vi "Saccade.vi"() -> ()   [LabVIEW 2012]
uses:
  <vilib>/Platform/TimedLoop/XDataNode/timing_clust.ctl
  <vilib>/Platform/TimedLoop/XDataNode/nitl_modes.ctl
  <vilib>/Platform/TimedLoop/XDataNode/wakeup.ctl
  <vilib>/DAQmx/write.llb/DAQmx Write (Analog DBL 1Chan 1Samp).vi
  <vilib>/DAQmx/miscellaneous.llb/DAQmx Fill In Error Info.vi
  SubVIs/VariablesToString_String.vi
  SubVIs/VariablesToString_Scalar.vi
  <vilib>/Platform/TimedLoop/XDataNode/XDataNode.xnode
  <vilib>/Platform/TimedLoop/XDataNode/XDNodeRunTimeDep.lvlib
  <vilib>/nisyscfg/nisyscfg.lvlib
  <vilib>/DAQmx/write.llb/DAQmx Write (Digital 1D Bool NChan 1Samp 1Line).vi
panel:
  in  "WfFlag":bool=TRUE
  out "WfGraph":cluster{dbl, dbl, dbl[][]}(graph)={-0.35, 0.04, array2x7714[15428 elements]}
  in  "SAFlag":bool
  in  "ElecStimSettings":T1={"TL"=200.0, "Freq"=200.0, "Dur"=0.2, "Amp"=10.0, "TD"=0.0, "DState"=enum."Ground", "TL2"=200.0, "Freq2"=200.0, "Dur2"=0.2, "Amp2"=10.0, "TD2"=0.0} {"Amp2" min=0.0 max=100.0 step=5.0; "Freq2" min=25.0 max=500.0 step=25.0; "Amp" min=0.0 max=100.0 step=5.0; "Freq" min=25.0 max=500.0 step=25.0}
  out "TrialStatus":T2={"TrialState"=enum."Initialize", "InitializeState"=enum."0", "FinalizeState"=enum."0", "HandsStatus"=enum."Both Hands On", "StimType"=enum."Photic", "Outcome"=enum."Abort", "AbortReason"=enum."Timed Out", "AbortLocation"=enum."Acq Stimulus"}
  out "GetHostTimeVI":path=path "E:/Code/Tasks/SubVIs/GetHostTime.vi"
  out "RunProgramVI":path=path "E:/Code/Tasks/SubVIs/RunProgram.vi"
  out "StopRecording":bool
  out "SaccadeFolder":path=path "E:/Code/Tasks/Saccade/Saccade_v2.0"
  out "CerebusFolder":string
  out "Recording?":bool
  out "AutoCentraVI":path=path "E:/Code/Tasks/SubVIs/AutoCentral.vi"
  out "TaskType":string="Saccade.vi"
  out "DatabaseUDL":path=path "E:/Data/Setup1_Database.udl"
  in  "Database":T3={"ExperimentDate"=timestamp(-9593222400 s since 1904-01-01), "ImplantDate"=timestamp(-9593222400 s since 1904-01-01), "CerebusFolder"="", "Experimenter"="", "PatientNumber"="", "DominantHand"="", "DeviceType"="", "DeviceSerial"="", "DeviceHemisphere"="", "DeviceRegion"="", "TaskType"="", "TaskComments"="", "RecordingComments"="", "GeneralObservations"=""}
  out "RemotePort":u16=9500
  out "RemoteIP":u32=2607134730
  out "UDPRef":refnum<k16>
  in  "RandFlag":bool
  in  "PhoticBnds":enum16{"Full Field", "LR Quadrant"}(ring)=enum."LR Quadrant" caption="Photic Bounds"
  out "AbortCount":u64
  in  "PlotSaccades":bool=TRUE
  out "LastPhoticStimPresets":T4(radio)=enum."Selection 1" caption="Stimulus Position"
  out "EyeXY":dbl[](array[numeric])=[0.6988403336972048, 0.026813536037091617] caption="Eye Position (X/Y)" format="%#.1g"
  out "EyeStatus":T5={"Fixation"=enum."In", "Photic"=enum."Out", "Electric"=enum."Out"}
  in  "SetElec":bool
  in  "ElectrodeStr":string="16;17;18;19,20,26;27;28;29,30,36;37;38;39;40;46;47;48;49;50;56;57;58;59;60;\r16;17;18;19;20;26;27;28;29;30;36;37;38;39;40;46;47;48;49,50,56;57;58;59,60,\r"
  out "ElectricArray":dbl[][](array[numeric])
  out "PhoticArray":dbl[][](array[numeric])
  in  "RandPhotic":bool
  out "Finished Late? [i-1]":bool
  out "ExpTime":u32 caption="Timer (min)" max=48 step=1
  out "Time/Date":timestamp=timestamp(3443552991.074658 s since 1904-01-01) format="%<%X\n%m/%d/%Y>T"
  out "LoopPeriod":u64=2
  out "LoopCount":u64=29507
  in  "StimSwitchSettings":T6={"ElecStimMode"=enum."Manual", "ElecPerc"=0.1}
  out "Damage Plot":cluster{"Y":dbl[], "Y":dbl[]}[](graph)=[{"Y"=[50.0], "Y"=[2.4999999999999996]}, {"Y"=[100.0, 0.0], "Y"=[0.0, 5.0]}] caption="Elec Curve"
  out "Current Electrode":i32=19 caption="Electrode"
  in  "RecordsSelection":string(combo)
  out "ExperimentDate":timestamp
  out "StimTypeBigIndicator":enum32{"---", "Photic", "Electric"}(ring)=enum."Photic" caption="Stimulation Type"
  out "MATLABCom":string="LV.ID='DrawPStim';LV.StimX=4.00;LV.StimY=0.00;LV.Radius=0.15;LV.Intensity=0.10;"
  out "LEDs":T7
  in  "ArrayReset":bool
  in  "Elec Indicators":T8={"Pulse Current"=250.0, "Pulse Charge"=50.0, "Pulse Charge Density"=2.4999999999999996, "SurfaceArea"=2000.0, "PhaseDuration"=0.2} {"PhaseDuration" format="%.4g"; "SurfaceArea" format="%.4g"; "Pulse Charge Density" format="%.4g"; "Pulse Charge" format="%.4g"; "Pulse Current" format="%.4g"}
  in  "Electrodes":T9={"Mixed Checkbox"=enum."False", "Mixed Checkbox 2"=enum."False", "Mixed Checkbox 3"=enum."False", "Mixed Checkbox 4"=enum."False", "Mixed Checkbox 5"=enum."False", "Mixed Checkbox 6"=enum."False", "Mixed Checkbox 7"=enum."False", "Mixed Checkbox 8"=enum."False", "Mixed Checkbox 9"=enum."False", "Mixed Checkbox 10"=enum."False", "Mixed Checkbox 11"=enum."False", "Mixed Checkbox 12"=enum."False", "Mixed Checkbox 13"=enum."False", "Mixed Checkbox 14"=enum."False", "Mixed Checkbox 15"=enum."False", "Mixed Checkbox 16"=enum."Mixed", "Mixed Checkbox 17"=enum."Mixed", "Mixed Checkbox 18"=enum."Mixed", "Mixed Checkbox 19"=enum."True", "Mixed Checkbox 20"=enum."True", "Mixed Checkbox 21"=enum."False", "Mixed Checkbox 22"=enum."False", "Mixed Checkbox 23"=enum."False", "Mixed Checkbox 24"=enum."False", "Mixed Checkbox 25"=enum."False", "Mixed Checkbox 26"=enum."Mixed", "Mixed Checkbox 27"=enum."Mixed", "Mixed Checkbox 28"=enum."Mixed", "Mixed Checkbox 29"=enum."True", "Mixed Checkbox 30"=enum."True", "Mixed Checkbox 31"=enum."False", "Mixed Checkbox 32"=enum."False", "Mixed Checkbox 33"=enum."False", "Mixed Checkbox 34"=enum."False", "Mixed Checkbox 35"=enum."False", "Mixed Checkbox 36"=enum."Mixed", "Mixed Checkbox 37"=enum."Mixed", "Mixed Checkbox 38"=enum."Mixed", "Mixed Checkbox 39"=enum."Mixed", "Mixed Checkbox 40"=enum."Mixed", "Mixed Checkbox 41"=enum."False", "Mixed Checkbox 42"=enum."False", "Mixed Checkbox 43"=enum."False", "Mixed Checkbox 44"=enum."False", "Mixed Checkbox 45"=enum."False", "Mixed Checkbox 46"=enum."Mixed", "Mixed Checkbox 47"=enum."Mixed", "Mixed Checkbox 48"=enum."Mixed", "Mixed Checkbox 49"=enum."Mixed", "Mixed Checkbox 50"=enum."Mixed", "Mixed Checkbox 51"=enum."False", "Mixed Checkbox 52"=enum."False", "Mixed Checkbox 53"=enum."False", "Mixed Checkbox 54"=enum."False", "Mixed Checkbox 55"=enum."False", "Mixed Checkbox 56"=enum."Mixed", "Mixed Checkbox 57"=enum."Mixed", "Mixed Checkbox 58"=enum."Mixed", "Mixed Checkbox 59"=enum."Mixed", "Mixed Checkbox 60"=enum."Mixed", "Mixed Checkbox 61"=enum."False", "Mixed Checkbox 62"=enum."False", "Mixed Checkbox 63"=enum."False", "Mixed Checkbox 64"=enum."False", "Mixed Checkbox 65"=enum."False", "Mixed Checkbox 66"=enum."False", "Mixed Checkbox 67"=enum."False", "Mixed Checkbox 68"=enum."False", "Mixed Checkbox 69"=enum."False", "Mixed Checkbox 70"=enum."False", "Mixed Checkbox 71"=enum."False", "Mixed Checkbox 72"=enum."False", "Mixed Checkbox 73"=enum."False", "Mixed Checkbox 74"=enum."False", "Mixed Checkbox 75"=enum."False", "Mixed Checkbox 76"=enum."False", "Mixed Checkbox 77"=enum."False", "Mixed Checkbox 78"=enum."False", "Mixed Checkbox 79"=enum."False", "Mixed Checkbox 80"=enum."False", "Mixed Checkbox 81"=enum."False", "Mixed Checkbox 82"=enum."False", "Mixed Checkbox 83"=enum."False", "Mixed Checkbox 84"=enum."False", "Mixed Checkbox 85"=enum."False", "Mixed Checkbox 86"=enum."False", "Mixed Checkbox 87"=enum."False", "Mixed Checkbox 88"=enum."False", "Mixed Checkbox 89"=enum."False", "Mixed Checkbox 90"=enum."False", "Mixed Checkbox 91"=enum."False", "Mixed Checkbox 92"=enum."False", "Mixed Checkbox 93"=enum."False", "Mixed Checkbox 94"=enum."False", "Mixed Checkbox 95"=enum."False", "Mixed Checkbox 96"=enum."False", "Mixed Checkbox 97"=enum."False", "Mixed Checkbox 98"=enum."False", "Mixed Checkbox 99"=enum."False", "Mixed Checkbox 100"=enum."False"}
  in  "StimButton":bool
  in  "PauseControls":T10={"Stimulate"=FALSE, "StimLoad"=FALSE, "Fixate"=FALSE, "PauseType"=FALSE, "FixationTime"=500.0}
  in  "Global Controls":T11={"Stop"=FALSE, "Pause"=FALSE, "TrackEyes"=TRUE, "MonHands"=FALSE, "Comment"=FALSE, "ElecReset"=FALSE, "PhoticReset"=FALSE}
  in  "Timers":T12={"ST"={"AFD"=2000, "SD"=1000, "HF"=2000, "HS"=1000, "BRD"=350, "FPD"=1000, "AS"=1000}, "RT"={"AFD"=0, "SD"=0, "HF"=300, "HS"=0, "BRD"=100, "AS"=0, "FPD"=100}, "AT"={"AFD"=2000, "SD"=300, "HF"=2105, "HS"=1000, "BRD"=282, "AS"=1000, "FPD"=907}} {"RT"."FPD" step=1; "RT"."AS" step=1; "RT"."SD" step=1; "RT"."AFD" step=1; "RT"."HF" step=1; "RT"."HS" step=1; "RT"."BRD" step=1; "AT"."FPD" max=1000 step=50; "AT"."AS" max=10000 step=100; "AT"."SD" max=10000 step=100; "AT"."AFD" max=10000 step=100; "AT"."HF" max=10000 step=50; "AT"."HS" max=10000 step=100; "AT"."BRD" max=1000 step=50; "ST"."FPD" step=1; "ST"."SD" step=1; "ST"."AFD" step=1; "ST"."HF" step=1; "ST"."HS" step=1; "ST"."BRD" step=1; "ST"."AS" step=1}
  in  "PhoticStimSettings":T13={"StimIntensity"=0.1, "StimRadius"=0.15, "StimX"=4.0, "StimY"=0.0, "BGnd"=0.0} caption="Photic Stimulus Settings" {"BGnd" format="%.2f"; "StimIntensity" format="%.3g"; "StimRadius" min=0.1 max=1.0 format="%.2g"; "StimY" format="%.2f"; "StimX" format="%.2f"}
  out "Stats":T14={"Photic"={"AcqStimulus"=7.0, "HoldStimulus"=0.0, "HoldFixation"=0.0, "Successful"=0.0, "Total"=7.0, "RemovedHands"=0.0}, "Electric"={"AcqStimulus"=2.0, "HoldStimulus"=0.0, "HoldFixation"=0.0, "Successful"=0.0, "Total"=2.0, "RemovedHands"=0.0}} {"Electric"."RemovedHands" min=0.0 format="%#.4g"; "Electric"."Total" min=0.0 format="%#.4g"; "Electric"."Successful" min=0.0 format="%#.4g"; "Electric"."HoldFixation" min=0.0 format="%#.4g"; "Electric"."HoldStimulus" min=0.0 format="%#.4g"; "Electric"."AcqStimulus" min=0.0 format="%#.4g"; "Photic"."RemovedHands" min=0.0 format="%#.4g"; "Photic"."Total" min=0.0 format="%#.4g"; "Photic"."Successful" min=0.0 format="%#.4g"; "Photic"."HoldFixation" min=0.0 format="%#.4g"; "Photic"."HoldStimulus" min=0.0 format="%#.4g"; "Photic"."AcqStimulus" min=0.0 format="%#.4g"}
  in  "PhoticStimPresets":T4(radio)=enum."Selection 1" caption="Stimulus Position"
  in  "EyeCalibration":T15={"Eye"={"OffsetX"=-0.6000000000000002, "OffsetY"=0.9000000000000005, "GainNegX"=5.279999999999999, "GainNegY"=4.1000000000000005, "GainPosX"=6.1, "GainPosY"=3.920000000000007, "RotNegX"=0.039999999999999994, "RotNegY"=0.0, "RotPosX"=-0.039999999999999994, "RotPosY"=0.12000000000000209}, "Fix"={"X"=0.0, "Y"=0.0, "R"=1.5}, "Photic"={"X"=4.0, "Y"=0.0, "R"=1.4999999999999998}, "Elec"={"X"=5.550000000000005, "Y"=-6.000000000000007, "R"=4.000000000000011}} caption="Eye Calibration" {"Elec"."X" min=-100.0 max=100.0 step=0.05 format="%.2f"; "Elec"."Y" min=-100.0 max=100.0 step=0.05 format="%.2f"; "Elec"."R" min=-100.0 max=100.0 step=0.05 format="%.2g"; "Photic"."X" min=-100.0 max=100.0 step=0.05 format="%.2f"; "Photic"."Y" min=-100.0 max=100.0 step=0.05 format="%.2f"; "Photic"."R" min=-100.0 max=100.0 step=0.05 format="%.2g"; "Fix"."X" min=-100.0 max=100.0 step=0.05 format="%.2f"; "Fix"."Y" min=-100.0 max=100.0 step=0.05 format="%.2f"; "Fix"."R" min=-100.0 max=100.0 step=0.05 format="%.2g"; "Eye"."RotPosY" min=-100.0 max=100.0 step=0.02 format="%.2g"; "Eye"."RotPosX" min=-100.0 max=100.0 step=0.02 format="%.2f"; "Eye"."RotNegY" min=-100.0 max=100.0 step=0.02 format="%.2g"; "Eye"."RotNegX" min=-100.0 max=100.0 step=0.02 format="%.2f"; "Eye"."GainPosY" min=-100.0 max=100.0 step=0.02 format="%.2g"; "Eye"."GainPosX" min=-100.0 max=100.0 step=0.02 format="%.2f"; "Eye"."GainNegY" min=-100.0 max=100.0 step=0.02 format="%.2g"; "Eye"."GainNegX" min=-100.0 max=100.0 step=0.02 format="%.2f"; "Eye"."OffsetY" min=-100.0 max=100.0 step=0.02 format="%.2g"; "Eye"."OffsetX" min=-100.0 max=100.0 step=0.02 format="%.2g"}
  out "Eye Graph":cluster{"Y":dbl[], "Y":dbl[]}[](graph)=[{"Y"=[0.6988403336972048], "Y"=[0.026813536037091617]}, {"Y"=[], "Y"=[]}, {"Y"=[0.0, 0.1879998503464564, 0.37303483074728216, 0.5521868290270169, 0.722630511152573, 0.8816778784387097, 1.0268206588930329, 1.155769864163684, 1.2664918882530225, 1.3572405786990294, 1.4265847744427302, 1.4734308760930328, 1.4970400926424072, 1.4970400926424072, 1.473430876093033, 1.4265847744427305, 1.3572405786990291, 1.2664918882530225, 1.155769864163684, 1.0268206588930333, 0.8816778784387098, 0.7226305111525728, 0.5521868290270172, 0.37303483074728283, 0.1879998503464568, 1.836909530733566e-16, -0.18799985034645644, -0.37303483074728183, -0.5521868290270169, -0.722630511152573, -0.881677878438709, -1.0268206588930326, -1.155769864163684, -1.266491888253023, -1.3572405786990296, -1.4265847744427302, -1.473430876093033, -1.4970400926424072, -1.4970400926424072, -1.473430876093033, -1.4265847744427305, -1.3572405786990298, -1.2664918882530225, -1.1557698641636844, -1.0268206588930333, -0.88167787843871, -0.7226305111525742, -0.5521868290270168, -0.37303483074728305, -0.18799985034645697, -3.673819061467132e-16], "Y"=[1.5, 1.4881720519717168, 1.4528747416929466, 1.3946647288323772, 1.3144600200657954, 1.2135254915624212, 1.0934529411321172, 0.9561359846230346, 0.8037401924684948, 0.638668937347609, 0.4635254915624212, 0.2810719718785871, 0.09418577929397029, -0.0941857792939701, -0.2810719718785869, -0.4635254915624207, -0.6386689373476091, -0.8037401924684953, -0.9561359846230346, -1.093452941132117, -1.213525491562421, -1.3144600200657954, -1.394664728832377, -1.4528747416929464, -1.4881720519717168, -1.5, -1.4881720519717168, -1.4528747416929468, -1.3946647288323772, -1.3144600200657952, -1.2135254915624216, -1.0934529411321177, -0.9561359846230343, -0.8037401924684945, -0.6386689373476082, -0.46352549156242134, -0.28107197187858696, -0.09418577929396982, 0.09418577929396925, 0.2810719718785864, 0.46352549156242084, 0.6386689373476078, 0.8037401924684952, 0.956135984623034, 1.0934529411321168, 1.213525491562421, 1.3144600200657948, 1.3946647288323772, 1.4528747416929464, 1.4881720519717168, 1.5]}, {"Y"=[4.0, 4.187999850346456, 4.373034830747282, 4.552186829027017, 4.722630511152573, 4.88167787843871, 5.026820658893033, 5.155769864163684, 5.2664918882530225, 5.357240578699029, 5.4265847744427305, 5.473430876093033, 5.497040092642408, 5.497040092642408, 5.473430876093033, 5.4265847744427305, 5.357240578699029, 5.2664918882530225, 5.155769864163684, 5.026820658893033, 4.88167787843871, 4.722630511152572, 4.552186829027017, 4.373034830747283, 4.187999850346457, 4.0, 3.8120001496535436, 3.6269651692527183, 3.4478131709729833, 3.277369488847427, 3.118322121561291, 2.9731793411069676, 2.844230135836316, 2.7335081117469775, 2.6427594213009704, 2.57341522555727, 2.526569123906967, 2.5029599073575928, 2.5029599073575928, 2.526569123906967, 2.5734152255572695, 2.6427594213009704, 2.7335081117469775, 2.844230135836316, 2.9731793411069667, 3.11832212156129, 3.277369488847426, 3.4478131709729833, 3.626965169252717, 3.812000149653543, 3.9999999999999996], "Y"=[1.4999999999999998, 1.4881720519717165, 1.4528747416929464, 1.394664728832377, 1.3144600200657952, 1.213525491562421, 1.0934529411321172, 0.9561359846230345, 0.8037401924684947, 0.6386689373476089, 0.4635254915624211, 0.28107197187858707, 0.09418577929397028, -0.09418577929397008, -0.28107197187858685, -0.4635254915624206, -0.638668937347609, -0.8037401924684952, -0.9561359846230345, -1.0934529411321168, -1.2135254915624207, -1.3144600200657952, -1.3946647288323768, -1.4528747416929462, -1.4881720519717165, -1.4999999999999998, -1.4881720519717165, -1.4528747416929466, -1.394664728832377, -1.314460020065795, -1.2135254915624214, -1.0934529411321174, -0.9561359846230342, -0.8037401924684944, -0.6386689373476081, -0.4635254915624213, -0.2810719718785869, -0.09418577929396979, 0.09418577929396924, 0.28107197187858635, 0.4635254915624208, 0.6386689373476077, 0.803740192468495, 0.9561359846230338, 1.0934529411321168, 1.2135254915624207, 1.3144600200657945, 1.394664728832377, 1.4528747416929462, 1.4881720519717165, 1.4999999999999998]}, {"Y"=[], "Y"=[]}, {"Y"=[5.550000000000005, 6.051332934257223, 6.544759548659427, 7.022498210738721, 7.477014696406871, 7.901141009169904, 8.288188423714766, 8.632052971103171, 8.927311702008074, 9.169308209864093, 9.35422606518063, 9.47914900291477, 9.542106913713102, 9.542106913713102, 9.47914900291477, 9.35422606518063, 9.169308209864093, 8.927311702008074, 8.632052971103171, 8.288188423714768, 7.901141009169905, 7.477014696406871, 7.022498210738721, 6.544759548659429, 6.051332934257225, 5.550000000000006, 5.048667065742786, 4.555240451340584, 4.077501789261289, 3.6229853035931385, 3.198858990830108, 2.8118115762852445, 2.4679470288968397, 2.172688297991935, 1.9306917901359162, 1.7457739348193808, 1.6208509970852396, 1.5578930862869083, 1.5578930862869083, 1.6208509970852396, 1.7457739348193804, 1.9306917901359157, 2.1726882979919364, 2.467947028896839, 2.8118115762852423, 3.1988589908301055, 3.6229853035931354, 4.07750178926129, 4.555240451340581, 5.0486670657427855, 5.550000000000004], "Y"=[-1.9999999999999964, -2.031541194742085, -2.1256673554854726, -2.2808940564469915, -2.4947732798245434, -2.763932022500209, -3.0841254903143533, -3.4503040410052415, -3.856692820084015, -4.296882833739712, -4.763932022500214, -5.250474741657106, -5.748837921882752, -6.251162078117261, -6.749525258342907, -7.236067977499799, -7.703117166260302, -8.143307179916, -8.549695958994773, -8.91587450968566, -9.236067977499804, -9.505226720175472, -9.719105943553021, -9.874332644514542, -9.968458805257928, -10.000000000000018, -9.96845880525793, -9.874332644514542, -9.719105943553023, -9.50522672017547, -9.236067977499808, -8.915874509685661, -8.549695958994771, -8.143307179915999, -7.7031171662603, -7.2360679774998005, -6.749525258342907, -6.251162078117261, -5.748837921882755, -5.250474741657108, -4.763932022500215, -4.296882833739716, -3.8566928200840143, -3.4503040410052432, -3.0841254903143547, -2.7639320225002093, -2.494773279824545, -2.2808940564469915, -2.125667355485473, -2.0315411947420854, -1.9999999999999964]}, {"Y"=[], "Y"=[]}, {"Y"=[], "Y"=[]}, {"Y"=[0.0], "Y"=[0.0]}, {"Y"=[], "Y"=[]}, {"Y"=[4.0], "Y"=[0.0]}, {"Y"=[], "Y"=[]}, {"Y"=[5.550000000000005], "Y"=[-6.000000000000007]}, {"Y"=[], "Y"=[]}, {"Y"=[], "Y"=[]}, {"Y"=[3.5, 7.5, 7.5, 3.5, 3.5], "Y"=[-5.0, -5.0, -7.0, -7.0, -5.0]}, {"Y"=[6.0, -1.1021457184401395e-15, 9.0, 8.314915792601582, 3.44415089128581, -1.6532185776602093e-15, 12.0, 11.086554390135442, 8.485281374238568, 4.59220118838108, -2.204291436880279e-15], "Y"=[0.0, -6.0, 0.0, -3.444150891285806, -8.31491579260158, -9.0, 0.0, -4.5922011883810745, -8.485281374238571, -11.08655439013544, -12.0]}]
  in  "Comments":string="Stimming the six groups of 9."
  out "ExpStartTime":u32=96660144
  # "Global Controls"
  # "Eye Tracking Graph"
  # "Trial Parameters"
  # "Electric Parameters"
  # "Database"
  # "Electrodes"
  # "1  2  3  4  5  6  7  8  9 10"
  # "0  1  2  3  4  5  6  7  8  9"
  # "0  1  2  3  4  5  6  7  8  9"
  # "Wire Bundle"
  # "Photic Parameters"
  # "1  2  3  4  5  6  7  8  9 10"
  # "Eye Calibration"
  # "Pulse Parameters"
  # "Status Panel"
  # "Damage Threshold"
  # "Statistics"
  # "Do not place ';' or '=' in the comment fields"
  # "Pause Controls"
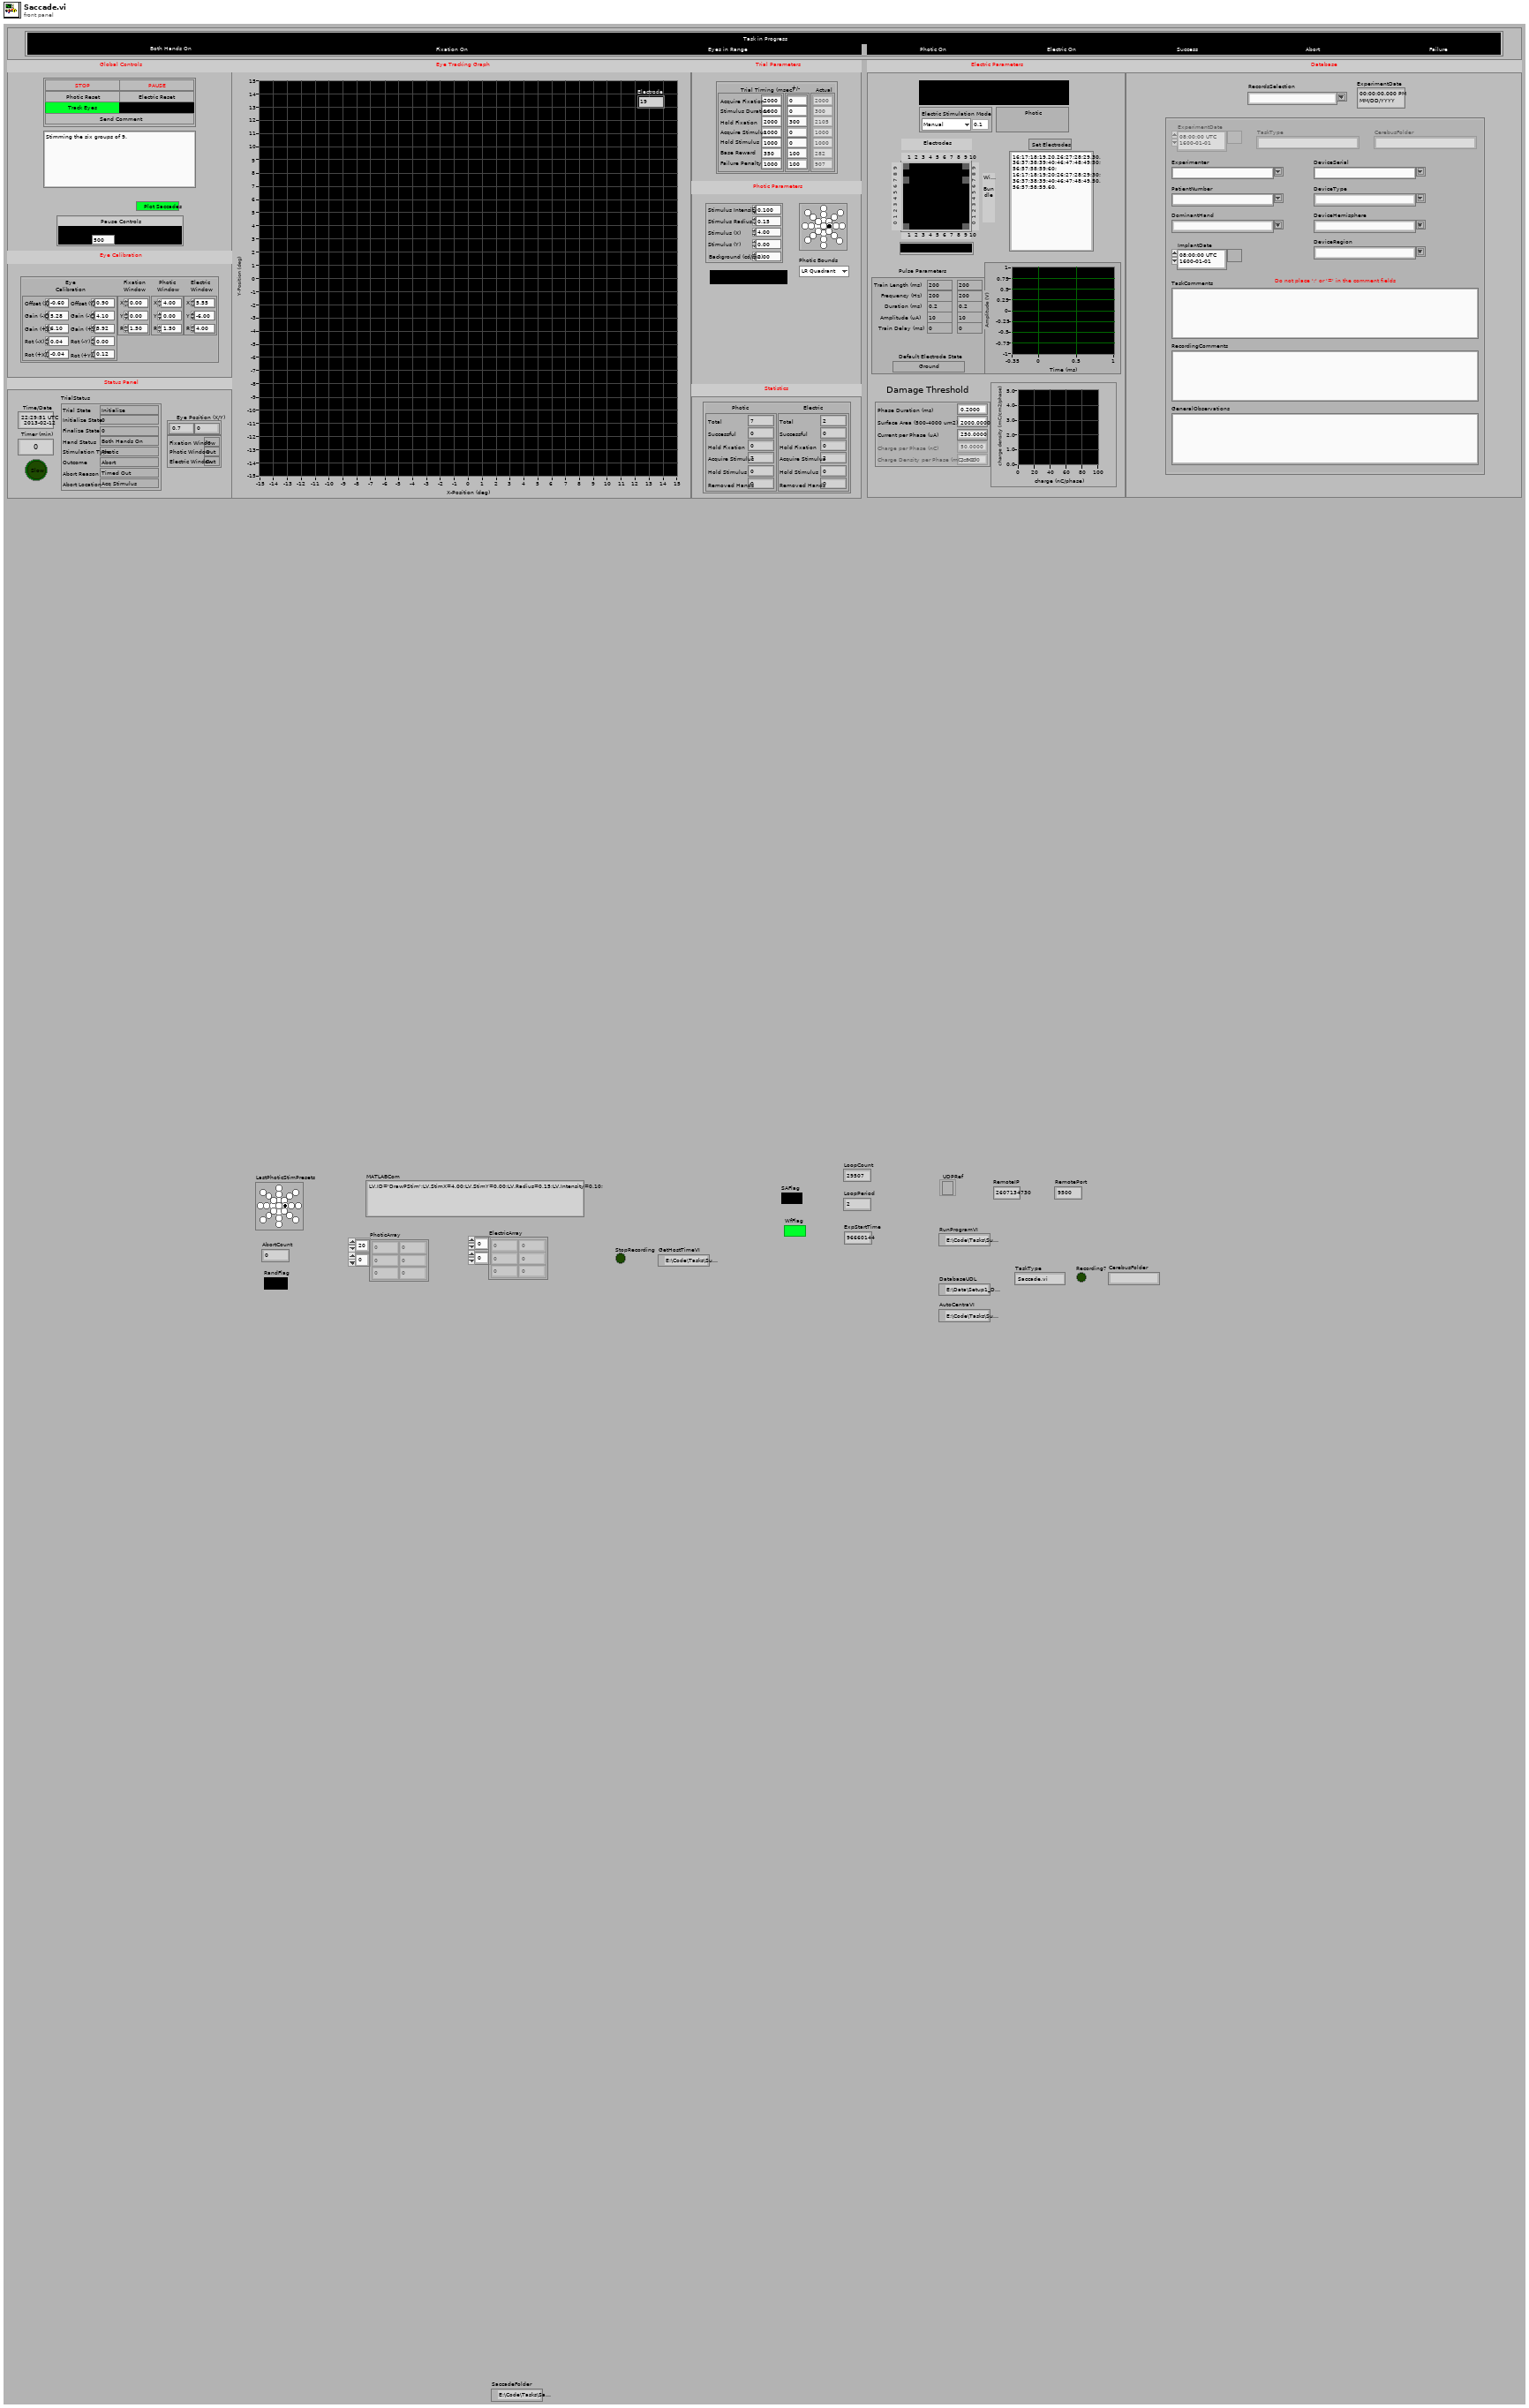
[diagram p1: front panel]
types:
  T1 = cluster{"TL":dbl, "Freq":dbl, "Dur":dbl, "Amp":dbl, "TD":dbl, "DState":enum16{"Ground", "Zero Current", "Open"}, "TL2":dbl, "Freq2":dbl, "Dur2":dbl, "Amp2":dbl, "TD2":dbl}
  T2 = cluster{"TrialState":enum32{"Initialize", "Acquire Fixation", "Visual Stimuli", "Finalize"}, "InitializeState":enum32{"0", "1", "2", "3", "4", "5", "6", "7", "8", "9", "10"}, "FinalizeState":enum32{"0", "1", "2", "3", "4", "5", "6", "7", "8", "9", "10"}, "HandsStatus":enum32{"Both Hands Off", "Left Hand Off", "Right Hand Off", "Both Hands On"}, "StimType":enum32{"---", "Photic", "Electric"}, "Outcome":enum32{"---", "Success", "Abort"}, "AbortReason":enum32{"---", "Looked Away", "Removed Hands", "Timed Out"}, "AbortLocation":enum32{"---", "Visual Stimuli", "Hold Fixation", "Acq Stimulus", "Hold Stimulus"}}
  T3 = cluster{"ExperimentDate":timestamp, "ImplantDate":timestamp, "CerebusFolder":string, "Experimenter":string, "PatientNumber":string, "DominantHand":string, "DeviceType":string, "DeviceSerial":string, "DeviceHemisphere":string, "DeviceRegion":string, "TaskType":string, "TaskComments":string, "RecordingComments":string, "GeneralObservations":string}
  T4 = enum32{"Selection 0", "Selection 1", "Selection 2", "Selection 3", "Selection 4", "Selection 5", "Selection 6", "Selection 7", "Selection 8", "Selection 9", "Selection 10", "Selection 11", "Selection 12", "Selection 13", "Selection 14", "Selection 15", "Selection 16", "Selection 17", "Selection 18", "Selection 19", "Selection 20", "Selection 21", "Selection 22", "Selection 23", "Selection 24"}
  T5 = cluster{"Fixation":enum16{"In", "Out"}, "Photic":enum16{"In", "Out"}, "Electric":enum16{"In", "Out"}}
  T6 = cluster{"ElecStimMode":enum16{"Continuous", "Manual"}, "ElecPerc":dbl}
  T7 = cluster{"InRange":bool, "TaskInProgress":bool, "Fixation":bool, "PStim":bool, "Success":bool, "Failure":bool, "Abort":bool, "HandsReady":bool, "RightHand":bool, "LeftHand":bool, "EStim":bool}
  T8 = cluster{"Pulse Current":dbl, "Pulse Charge":dbl, "Pulse Charge Density":dbl, "SurfaceArea":dbl, "PhaseDuration":dbl}
  T9 = cluster{"Mixed Checkbox":enum8{"False", "True", "Mixed"}, "Mixed Checkbox 2":enum8{"False", "True", "Mixed"}, "Mixed Checkbox 3":enum8{"False", "True", "Mixed"}, "Mixed Checkbox 4":enum8{"False", "True", "Mixed"}, "Mixed Checkbox 5":enum8{"False", "True", "Mixed"}, "Mixed Checkbox 6":enum8{"False", "True", "Mixed"}, "Mixed Checkbox 7":enum8{"False", "True", "Mixed"}, "Mixed Checkbox 8":enum8{"False", "True", "Mixed"}, "Mixed Checkbox 9":enum8{"False", "True", "Mixed"}, "Mixed Checkbox 10":enum8{"False", "True", "Mixed"}, "Mixed Checkbox 11":enum8{"False", "True", "Mixed"}, "Mixed Checkbox 12":enum8{"False", "True", "Mixed"}, "Mixed Checkbox 13":enum8{"False", "True", "Mixed"}, "Mixed Checkbox 14":enum8{"False", "True", "Mixed"}, "Mixed Checkbox 15":enum8{"False", "True", "Mixed"}, "Mixed Checkbox 16":enum8{"False", "True", "Mixed"}, "Mixed Checkbox 17":enum8{"False", "True", "Mixed"}, "Mixed Checkbox 18":enum8{"False", "True", "Mixed"}, "Mixed Checkbox 19":enum8{"False", "True", "Mixed"}, "Mixed Checkbox 20":enum8{"False", "True", "Mixed"}, "Mixed Checkbox 21":enum8{"False", "True", "Mixed"}, "Mixed Checkbox 22":enum8{"False", "True", "Mixed"}, "Mixed Checkbox 23":enum8{"False", "True", "Mixed"}, "Mixed Checkbox 24":enum8{"False", "True", "Mixed"}, "Mixed Checkbox 25":enum8{"False", "True", "Mixed"}, "Mixed Checkbox 26":enum8{"False", "True", "Mixed"}, "Mixed Checkbox 27":enum8{"False", "True", "Mixed"}, "Mixed Checkbox 28":enum8{"False", "True", "Mixed"}, "Mixed Checkbox 29":enum8{"False", "True", "Mixed"}, "Mixed Checkbox 30":enum8{"False", "True", "Mixed"}, "Mixed Checkbox 31":enum8{"False", "True", "Mixed"}, "Mixed Checkbox 32":enum8{"False", "True", "Mixed"}, "Mixed Checkbox 33":enum8{"False", "True", "Mixed"}, "Mixed Checkbox 34":enum8{"False", "True", "Mixed"}, "Mixed Checkbox 35":enum8{"False", "True", "Mixed"}, "Mixed Checkbox 36":enum8{"False", "True", "Mixed"}, "Mixed Checkbox 37":enum8{"False", "True", "Mixed"}, "Mixed Checkbox 38":enum8{"False", "True", "Mixed"}, "Mixed Checkbox 39":enum8{"False", "True", "Mixed"}, "Mixed Checkbox 40":enum8{"False", "True", "Mixed"}, "Mixed Checkbox 41":enum8{"False", "True", "Mixed"}, "Mixed Checkbox 42":enum8{"False", "True", "Mixed"}, "Mixed Checkbox 43":enum8{"False", "True", "Mixed"}, "Mixed Checkbox 44":enum8{"False", "True", "Mixed"}, "Mixed Checkbox 45":enum8{"False", "True", "Mixed"}, "Mixed Checkbox 46":enum8{"False", "True", "Mixed"}, "Mixed Checkbox 47":enum8{"False", "True", "Mixed"}, "Mixed Checkbox 48":enum8{"False", "True", "Mixed"}, "Mixed Checkbox 49":enum8{"False", "True", "Mixed"}, "Mixed Checkbox 50":enum8{"False", "True", "Mixed"}, "Mixed Checkbox 51":enum8{"False", "True", "Mixed"}, "Mixed Checkbox 52":enum8{"False", "True", "Mixed"}, "Mixed Checkbox 53":enum8{"False", "True", "Mixed"}, "Mixed Checkbox 54":enum8{"False", "True", "Mixed"}, "Mixed Checkbox 55":enum8{"False", "True", "Mixed"}, "Mixed Checkbox 56":enum8{"False", "True", "Mixed"}, "Mixed Checkbox 57":enum8{"False", "True", "Mixed"}, "Mixed Checkbox 58":enum8{"False", "True", "Mixed"}, "Mixed Checkbox 59":enum8{"False", "True", "Mixed"}, "Mixed Checkbox 60":enum8{"False", "True", "Mixed"}, "Mixed Checkbox 61":enum8{"False", "True", "Mixed"}, "Mixed Checkbox 62":enum8{"False", "True", "Mixed"}, "Mixed Checkbox 63":enum8{"False", "True", "Mixed"}, "Mixed Checkbox 64":enum8{"False", "True", "Mixed"}, "Mixed Checkbox 65":enum8{"False", "True", "Mixed"}, "Mixed Checkbox 66":enum8{"False", "True", "Mixed"}, "Mixed Checkbox 67":enum8{"False", "True", "Mixed"}, "Mixed Checkbox 68":enum8{"False", "True", "Mixed"}, "Mixed Checkbox 69":enum8{"False", "True", "Mixed"}, "Mixed Checkbox 70":enum8{"False", "True", "Mixed"}, "Mixed Checkbox 71":enum8{"False", "True", "Mixed"}, "Mixed Checkbox 72":enum8{"False", "True", "Mixed"}, "Mixed Checkbox 73":enum8{"False", "True", "Mixed"}, "Mixed Checkbox 74":enum8{"False", "True", "Mixed"}, "Mixed Checkbox 75":enum8{"False", "True", "Mixed"}, "Mixed Checkbox 76":enum8{"False", "True", "Mixed"}, "Mixed Checkbox 77":enum8{"False", "True", "Mixed"}, "Mixed Checkbox 78":enum8{"False", "True", "Mixed"}, "Mixed Checkbox 79":enum8{"False", "True", "Mixed"}, "Mixed Checkbox 80":enum8{"False", "True", "Mixed"}, "Mixed Checkbox 81":enum8{"False", "True", "Mixed"}, "Mixed Checkbox 82":enum8{"False", "True", "Mixed"}, "Mixed Checkbox 83":enum8{"False", "True", "Mixed"}, "Mixed Checkbox 84":enum8{"False", "True", "Mixed"}, "Mixed Checkbox 85":enum8{"False", "True", "Mixed"}, "Mixed Checkbox 86":enum8{"False", "True", "Mixed"}, "Mixed Checkbox 87":enum8{"False", "True", "Mixed"}, "Mixed Checkbox 88":enum8{"False", "True", "Mixed"}, "Mixed Checkbox 89":enum8{"False", "True", "Mixed"}, "Mixed Checkbox 90":enum8{"False", "True", "Mixed"}, "Mixed Checkbox 91":enum8{"False", "True", "Mixed"}, "Mixed Checkbox 92":enum8{"False", "True", "Mixed"}, "Mixed Checkbox 93":enum8{"False", "True", "Mixed"}, "Mixed Checkbox 94":enum8{"False", "True", "Mixed"}, "Mixed Checkbox 95":enum8{"False", "True", "Mixed"}, "Mixed Checkbox 96":enum8{"False", "True", "Mixed"}, "Mixed Checkbox 97":enum8{"False", "True", "Mixed"}, "Mixed Checkbox 98":enum8{"False", "True", "Mixed"}, "Mixed Checkbox 99":enum8{"False", "True", "Mixed"}, "Mixed Checkbox 100":enum8{"False", "True", "Mixed"}}
  T10 = cluster{"Stimulate":bool, "StimLoad":bool, "Fixate":bool, "PauseType":bool, "FixationTime":dbl}
  T11 = cluster{"Stop":bool, "Pause":bool, "TrackEyes":bool, "MonHands":bool, "Comment":bool, "ElecReset":bool, "PhoticReset":bool}
  T12 = cluster{"ST":cluster{"AFD":u64, "SD":u64, "HF":u64, "HS":u64, "BRD":u64, "FPD":u64, "AS":u64}, "RT":cluster{"AFD":u64, "SD":u64, "HF":u64, "HS":u64, "BRD":u64, "AS":u64, "FPD":u64}, "AT":cluster{"AFD":u64, "SD":u64, "HF":u64, "HS":u64, "BRD":u64, "AS":u64, "FPD":u64}}
  T13 = cluster{"StimIntensity":dbl, "StimRadius":dbl, "StimX":dbl, "StimY":dbl, "BGnd":dbl}
  T14 = cluster{"Photic":cluster{"AcqStimulus":dbl, "HoldStimulus":dbl, "HoldFixation":dbl, "Successful":dbl, "Total":dbl, "RemovedHands":dbl}, "Electric":cluster{"AcqStimulus":dbl, "HoldStimulus":dbl, "HoldFixation":dbl, "Successful":dbl, "Total":dbl, "RemovedHands":dbl}}
  T15 = cluster{"Eye":cluster{"OffsetX":dbl, "OffsetY":dbl, "GainNegX":dbl, "GainNegY":dbl, "GainPosX":dbl, "GainPosY":dbl, "RotNegX":dbl, "RotNegY":dbl, "RotPosX":dbl, "RotPosY":dbl}, "Fix":cluster{"X":dbl, "Y":dbl, "R":dbl}, "Photic":cluster{"X":dbl, "Y":dbl, "R":dbl}, "Elec":cluster{"X":dbl, "Y":dbl, "R":dbl}}
  T16 = enum16{"Initialize", "String", "Start", "New Session", "Stop", "Resume", "Close"}
  T17 = enum16{"SaveConfiguration", "StartRecording", "StopRecording"}
  T18 = enum32{"Both Hands Off", "Left Hand Off", "Right Hand Off", "Both Hands On"}
  T19 = enum32{"---", "Looked Away", "Removed Hands", "Timed Out"}
  T20 = enum32{"---", "Visual Stimuli", "Hold Fixation", "Acq Stimulus", "Hold Stimulus"}
  T21 = enum32{"Initialize", "Acquire Fixation", "Visual Stimuli", "Finalize"}
  T22 = enum32{"0", "1", "2", "3", "4", "5", "6", "7", "8", "9", "10"}
  T23 = cluster{"AcqStimulus":dbl, "HoldStimulus":dbl, "HoldFixation":dbl, "Successful":dbl, "Total":dbl, "RemovedHands":dbl}
  T24 = typedef "XDNodeRunTimeDep.lvlib/timing_clust.ctl" = cluster{"Expected End [f-1]":u64, "Actual End [f-1]":u64, "Finished Late? [f-1]":bool, "Expected End [i-1]":u64, "Actual End [i-1]":u64, "Finished Late? [i-1]":bool, "Expected Start [i]":u64, "Actual Start [i]":u64, "Expected Start [f]":u64, "Actual Start [f]":u64, "Source Name":string, "Structure Name":string, "Period":i64, "Deadline":i64, "Offset":i64, "Start":i64, "Priority":i32, "Timeout":i32, "Mode":T25, "Wakeup Reason":T26, "Error":errorcluster, "Source Type":string, "Secondary Source Type":string, "Global End Time":u64, "Global Start Time":u64, "Frame Duration":u64, "Iteration Duration":u64, "Assigned CPU":i32, "I/O Scan Engine Mode":u32}
  T25 = typedef "XDNodeRunTimeDep.lvlib/nitl_modes.ctl" = enum32{"No Change", "Process missed periods, maintain original phase", "Discard missed periods, maintain original phase", "Process missed periods, ignore original phase", "Discard missed periods, ignore original phase"}
  T26 = typedef "XDNodeRunTimeDep.lvlib/wakeup.ctl" = enum32{"Normal", "Aborted", "Asynchronous wakeup", "Timing source error", "Timed loop error", "Timeout"}
  T27 = cluster{"Pulse Current":bool, "Pulse Charge":bool, "Pulse Charge Density":bool, "SurfaceArea":bool, "PhaseDuration":bool}
  T28 = cluster{"[0]":i32, "[1]":i32, "[2]":i32, "[3]":i32, "[4]":i32, "[5]":i32, "[6]":i32, "[7]":i32, "[8]":i32, "[9]":i32, "[10]":i32, "[11]":i32, "[12]":i32, "[13]":i32, "[14]":i32, "[15]":i32, "[16]":i32, "[17]":i32, "[18]":i32, "[19]":i32, "[20]":i32, "[21]":i32, "[22]":i32, "[23]":i32, "[24]":i32, "[25]":i32, "[26]":i32, "[27]":i32, "[28]":i32, "[29]":i32, "[30]":i32, "[31]":i32, "[32]":i32, "[33]":i32, "[34]":i32, "[35]":i32, "[36]":i32, "[37]":i32, "[38]":i32, "[39]":i32, "[40]":i32, "[41]":i32, "[42]":i32, "[43]":i32, "[44]":i32, "[45]":i32, "[46]":i32, "[47]":i32, "[48]":i32, "[49]":i32, "[50]":i32, "[51]":i32, "[52]":i32, "[53]":i32, "[54]":i32, "[55]":i32, "[56]":i32, "[57]":i32, "[58]":i32, "[59]":i32, "[60]":i32, "[61]":i32, "[62]":i32, "[63]":i32, "[64]":i32, "[65]":i32, "[66]":i32, "[67]":i32, "[68]":i32, "[69]":i32, "[70]":i32, "[71]":i32, "[72]":i32, "[73]":i32, "[74]":i32, "[75]":i32, "[76]":i32, "[77]":i32, "[78]":i32, "[79]":i32, "[80]":i32, "[81]":i32, "[82]":i32, "[83]":i32, "[84]":i32, "[85]":i32, "[86]":i32, "[87]":i32, "[88]":i32, "[89]":i32, "[90]":i32, "[91]":i32, "[92]":i32, "[93]":i32, "[94]":i32, "[95]":i32, "[96]":i32, "[97]":i32, "[98]":i32, "[99]":i32}
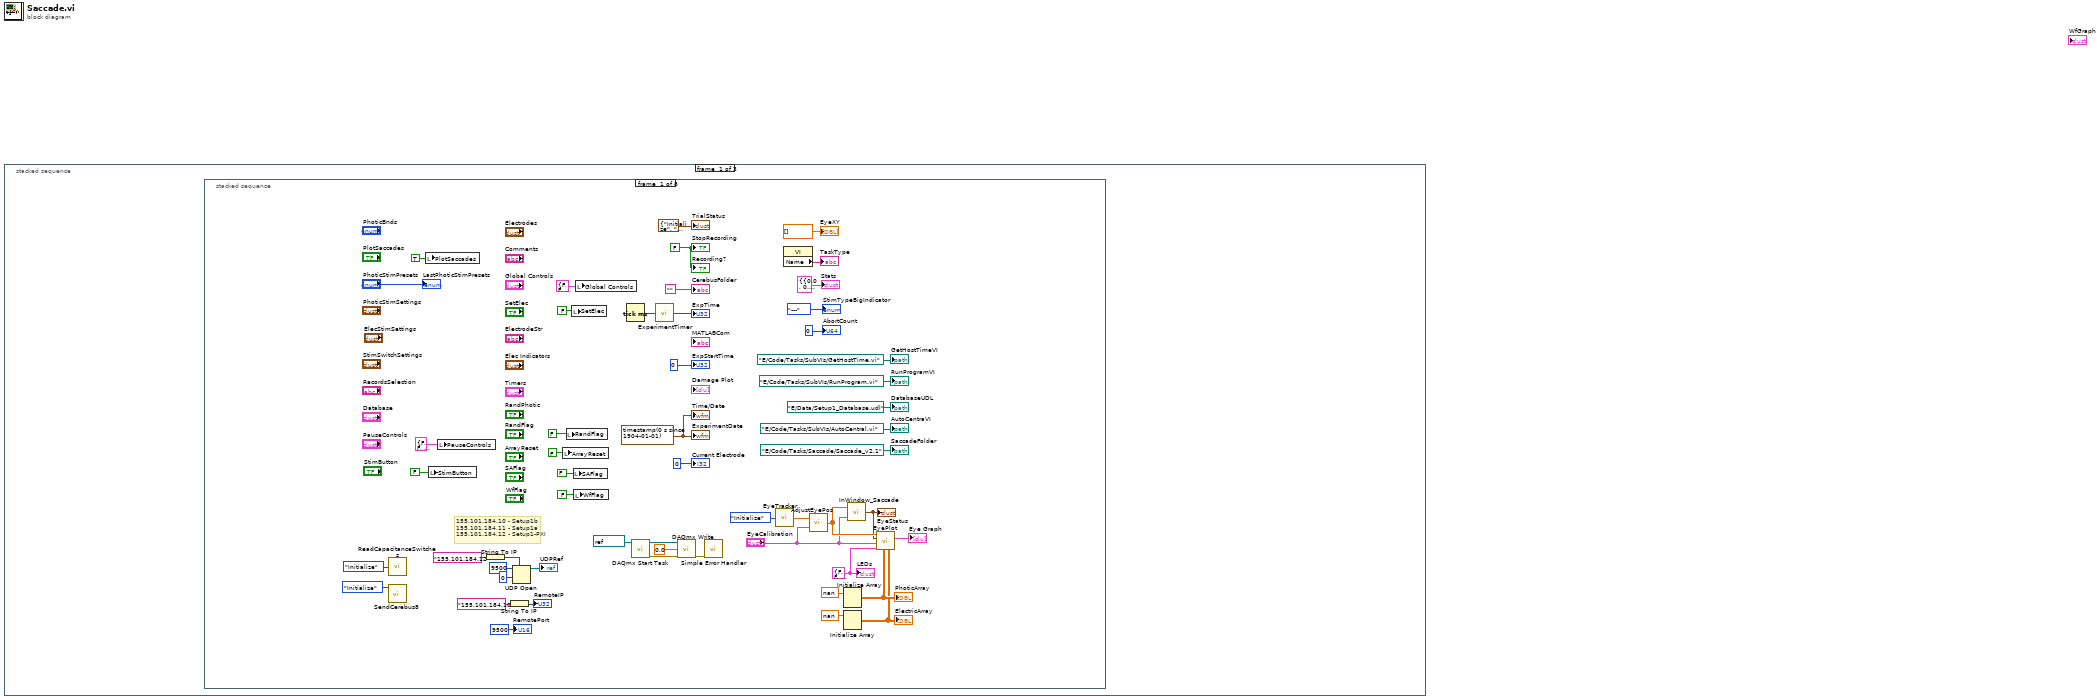
[diagram p0: block diagram]
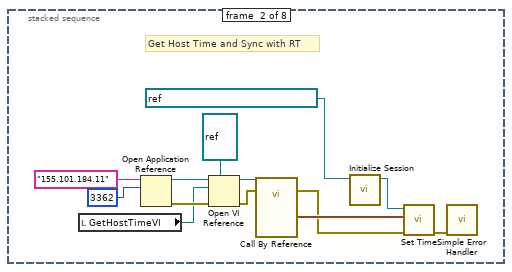
[diagram p2: hidden frame]
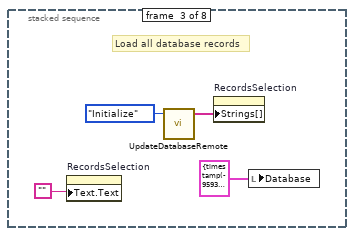
[diagram p3: hidden frame]
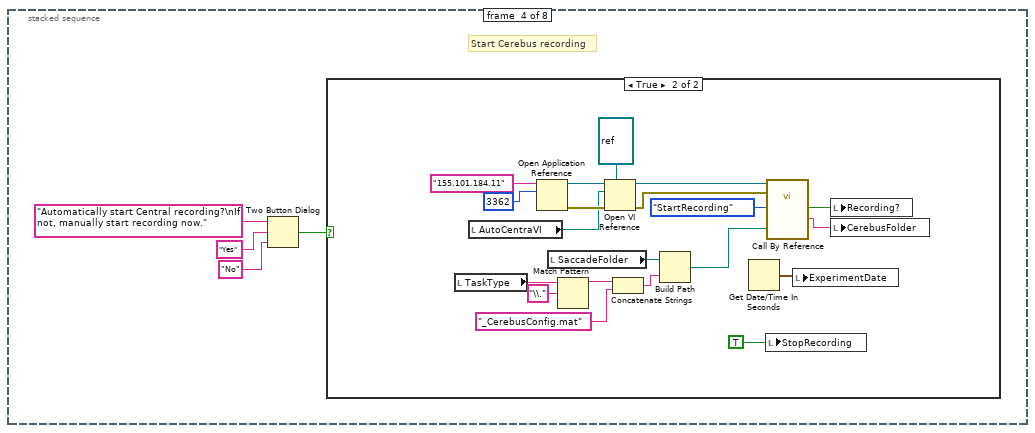
[diagram p4: hidden frame]
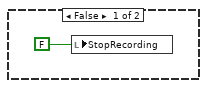
[diagram p5: hidden frame]
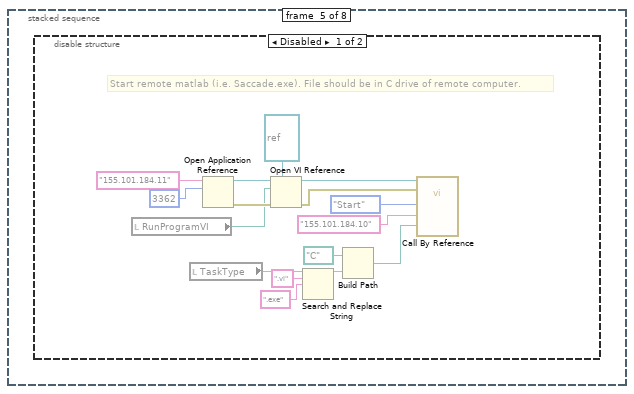
[diagram p6: hidden frame]
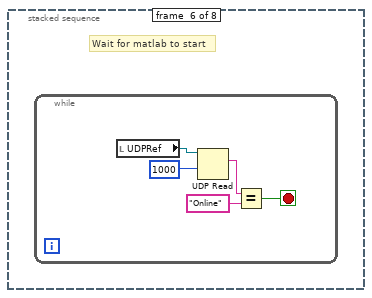
[diagram p8: hidden frame]
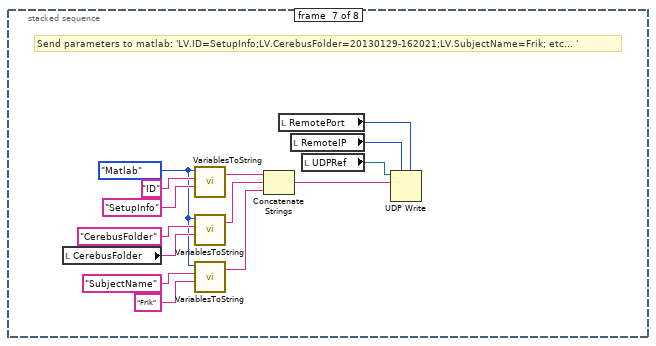
[diagram p9: hidden frame]
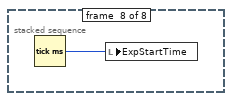
[diagram p10: hidden frame]
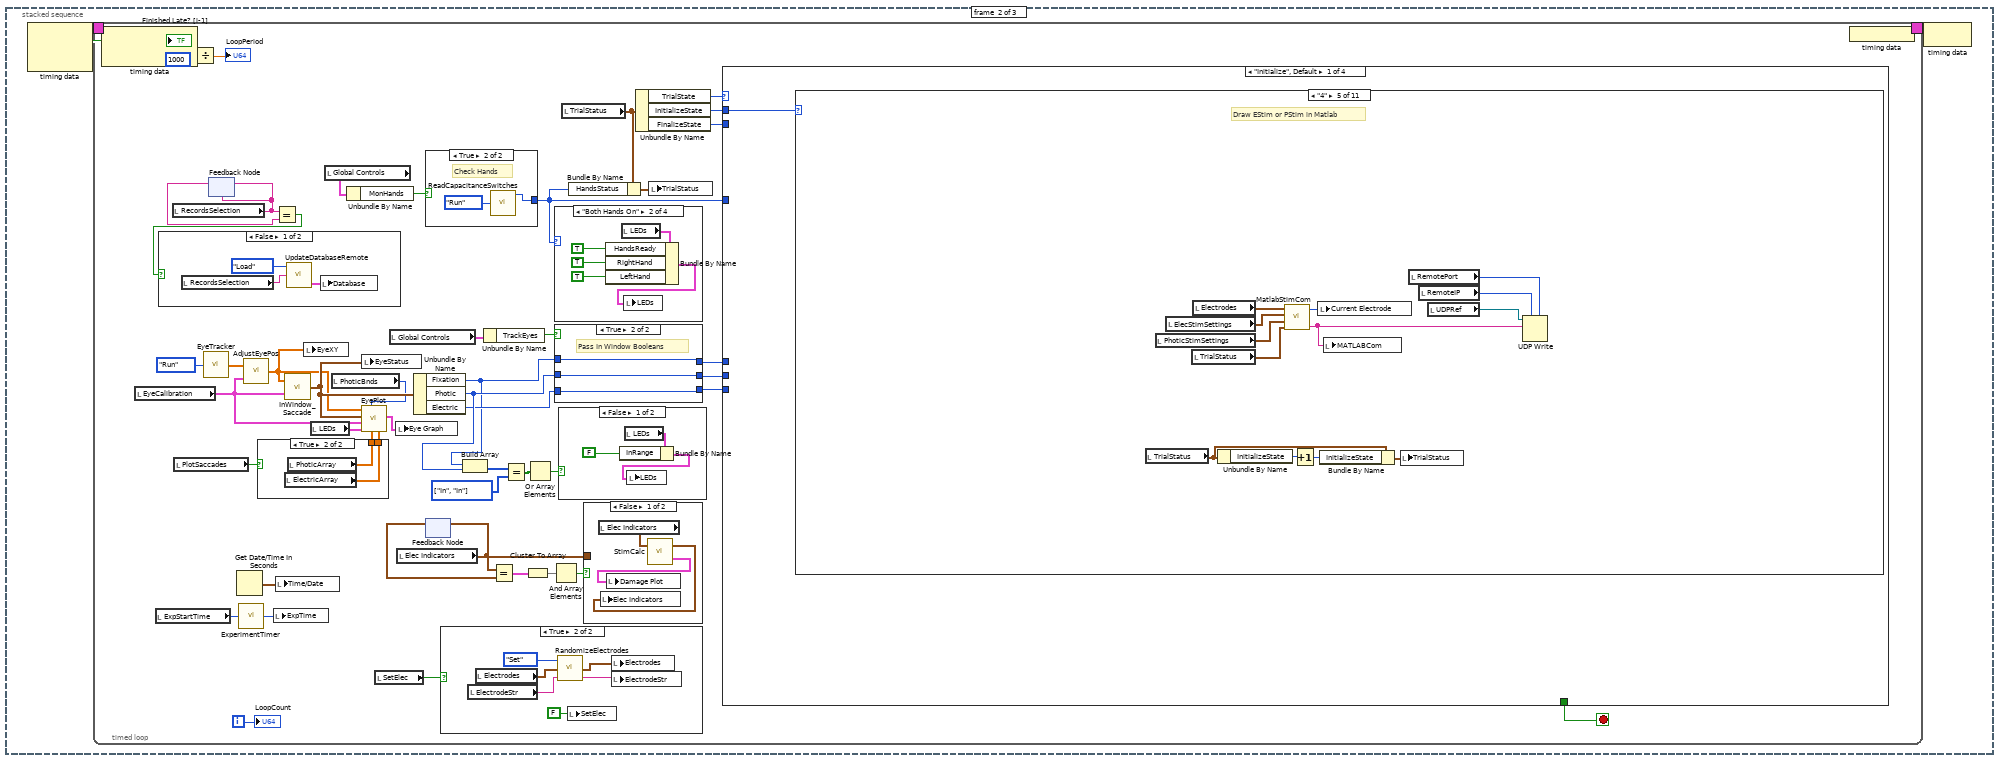
[diagram p11: hidden frame]
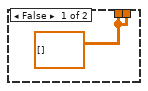
[diagram p12: hidden frame]
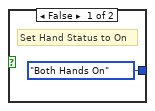
[diagram p14: hidden frame]
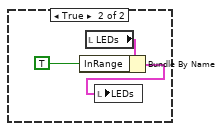
[diagram p15: hidden frame]
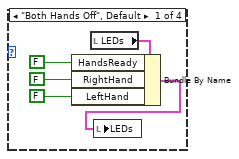
[diagram p16: hidden frame]
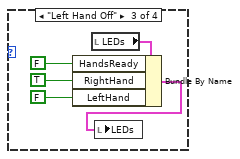
[diagram p17: hidden frame]
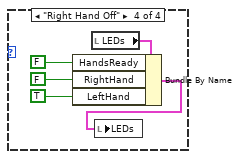
[diagram p18: hidden frame]
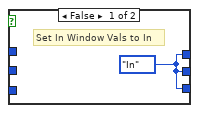
[diagram p19: hidden frame]
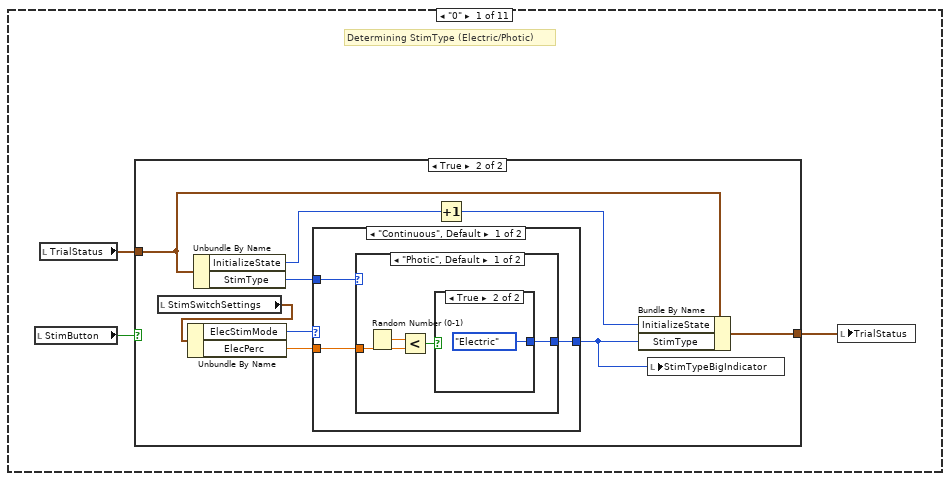
[diagram p20: hidden frame]
diagram:
  n1 = stacked-sequence {
    frame #0 {
      n2 = stacked-sequence {
        frame #0 {
          w6 = FALSE ("StopRecording")
          w9 = timestamp(0 s since 1904-01-01)
          w38 = T7 {"InRange"=FALSE, "TaskInProgress"=FALSE, "Fixation"=FALSE, "PStim"=FALSE, "Success"=FALSE, "Failure"=FALSE, "Abort"=FALSE, "HandsReady"=FALSE, "RightHand"=FALSE, "LeftHand"=FALSE, "EStim"=FALSE} ("LEDs")
          # "155.101.184.10 - Setup1b\n155.101.184.11 - Setup1a\n155.101.184.12 - Setup1-PXI"
          n3 = call "SendCerebus8.vi"("Mode"=T16."Initialize") -> ()  [unwired: 4 in]
          n4 = call "ReadCapacitanceSwitches.vi"("Mode"=enum32{"Initialize", "Run", "Close"}."Initialize") -> ()  [unwired: 3 out]
          n5 = local write "PlotSaccades"(TRUE ("PlotSaccades")) -> ()
          n6 = local write "StimButton"(FALSE ("Warning Watch")) -> ()
          n7 = local write "PauseControls"(T10 {"Stimulate"=FALSE, "StimLoad"=FALSE, "Fixate"=FALSE, "PauseType"=FALSE, "FixationTime"=500.0} ("PauseControls")) -> ()
          n8 = String To IP(1:"155.101.184.12" ("name")) -> (0:w19:u32)
          n9 = String To IP(1:"155.101.184.10" ("name")) -> (0:→"RemoteIP":u32)
          n10 = UDP Open(7:w19, 9:0 ("timeout ms (25000)"), 11:u16 9500 ("port")) -> (port=→"UDPRef":refnum<k16>)  [unwired: 2 in, 2 out]
          n11 = local write "ArrayReset"(FALSE ("Array Reset")) -> ()
          n12 = local write "RandFlag"(FALSE ("RandPhotic")) -> ()
          n13 = local write "SetElec"(FALSE ("SetElec")) -> ()
          n14 = local write "SAFlag"(FALSE ("Array Reset")) -> ()
          n15 = local write "WfFlag"(FALSE ("Array Reset")) -> ()
          n16 = local write "Global Controls"(T11 {"Stop"=FALSE, "Pause"=FALSE, "TrackEyes"=TRUE, "MonHands"=FALSE, "Comment"=FALSE, "ElecReset"=FALSE, "PhoticReset"=FALSE} ("Global Controls")) -> ()
          n17 = Tick Count (ms)() -> (millisecond timer value=w51:u32)
          n18 = call <vilib>:"DAQmx Start Task.vi"("task/channels in"=refnum<k21> "Juice") -> ("task out"=w41:refnum<k21>, "error out"=w40:errorcluster)  [unwired: 13 in]
          n19 = call "ExperimentTimer.vi"("Experiment Start Time"=w51) -> ("Exp Timer"=→"ExpTime":u32)
          n20 = call-poly <vilib>:"DAQmx Write.vi"("task/channels in"=w41, "data"=0.0, "error in"=w40) -> ("error out"=w39:errorcluster)  [unwired: 10 in, 2 out]
          n21 = call <vilib>:"Simple Error Handler.vi"("error in (no error)"=w39) -> ()  [unwired: 4 in, 5 out]
          n22 = call "EyeTracker.vi"("Mode"=enum16{"Initialize", "Run", "Close"}."Initialize") -> ("EyeXY"=w30:dbl[])
          n23 = property class="VI"() -> ("Name"=→"TaskType":string)  [unwired: 2 in, 2 out]
          n24 = call "AdjustEyePos.vi"("EyeCalibration"="EyeCalibration", "EyeXYIn"=w30) -> ("EyeXYOut"=w29:dbl[])
          n25 = Initialize Array(nan ("element")) -> (w25:dbl[][])  [unwired: 2 in]
          "PhoticArray" <- w25
          n26 = Initialize Array(nan ("element")) -> (w24:dbl[][])  [unwired: 2 in]
          "ElectricArray" <- w24
          n27 = call "InWindow_Saccade.vi"("EyeCalibration"="EyeCalibration", "EyeXY"=w29) -> ("EyeStatus"=w27:T5)
          "EyeStatus" <- w27
          n28 = call "EyePlot.vi"("ElectricArray"=w24, "PhoticArray"=w25, "LEDs"=w38, "EyeCalibration"="EyeCalibration", "EyeStatus"=w27, "EyeXY"=w29) -> ("EyeGraph"=→"Eye Graph":cluster{dbl[], dbl[]}[])  [unwired: 5 in]
          "ExpStartTime" <- u32 0 ("ExpStartTime")
          "Time/Date" <- w9
          "LEDs" <- w38
          "Stats" <- T14 {"Photic"={"AcqStimulus"=0.0, "HoldStimulus"=0.0, "HoldFixation"=0.0, "Successful"=0.0, "Total"=0.0, "RemovedHands"=0.0}, "Electric"={"AcqStimulus"=0.0, "HoldStimulus"=0.0, "HoldFixation"=0.0, "Successful"=0.0, "Total"=0.0, "RemovedHands"=0.0}} ("Stats")
          "StimTypeBigIndicator" <- enum32{"---", "Photic", "Electric"}."---" ("StimTypeBigIndicator")
          "ExperimentDate" <- w9
          "Current Electrode" <- 0 ("Current Electrode")
          "EyeXY" <- dbl[] [] ("EyeXY")
          "LastPhoticStimPresets" <- "PhoticStimPresets"
          "AbortCount" <- u64 0 ("BaseCount")
          "RemotePort" <- u16 9500 ("port or service name")
          "DatabaseUDL" <- path "E:/Data/Setup1_Database.udl" ("RemoteMatlab path")
          "AutoCentraVI" <- path "E:/Code/Tasks/SubVIs/AutoCentral.vi" ("RemoteMatlab path")
          "SaccadeFolder" <- path "E:/Code/Tasks/Saccade/Saccade_v2.1" ("base path")
          "StopRecording" <- w6
          "CerebusFolder" <- ""
          "Recording?" <- w6
          "RunProgramVI" <- path "E:/Code/Tasks/SubVIs/RunProgram.vi" ("RemoteMatlab path")
          "GetHostTimeVI" <- path "E:/Code/Tasks/SubVIs/GetHostTime.vi" ("RemoteMatlab path")
          "TrialStatus" <- T2 {"TrialState"=enum."Initialize", "InitializeState"=enum."0", "FinalizeState"=enum."0", "HandsStatus"=enum."Both Hands Off", "StimType"=enum."---", "Outcome"=enum."---", "AbortReason"=enum."---", "AbortLocation"=enum."---"} ("TrialStatus")
        }
        frame #1 {
          # "Get Host Time and Sync with RT"
          n29 = local read "GetHostTimeVI"() -> (w55:path)
          n30 = Open Application Reference(10:u16 3362 ("port number or service name (3363)"), 11:"155.101.184.11" ("machine name (\"\":  open local reference)")) -> (0:w62:errorcluster, 3:w65:refnum<vi>)  [unwired: 2 in]
          n31 = Open VI Reference(type specifier VI Refnum (for type only)=refnum<vi> refnum, application reference (local)=w65, vi path=w55, error in (no error)=w62) -> (vi reference=w63:refnum<vi>, error out=w61:errorcluster)  [unwired: 2 in]
          n32 = call-by-ref "?"(reference=w63, error in=w61) -> (error out=w59:errorcluster, "current time"=w60:timestamp)  [unwired: 1 in, 1 out]
          n33 = call <vilib>:"Initialize Session.vi"("target (localhost)"=refnum<k21> "Setup1-PXI (155.101.184.12)") -> ("session out"=w57:refnum<k21>)  [unwired: 9 in, 1 out]
          n34 = call <vilib>:"Set Time.vi"("error in (no error)"=w59, "time"=w60, "session in (localhost)"=w57) -> ("error out"=w58:errorcluster)  [unwired: 5 in, 3 out]
          n35 = call <vilib>:"Simple Error Handler.vi"("error in (no error)"=w58) -> ()  [unwired: 4 in, 5 out]
        }
        frame #2 {
          # "Load all database records"
          n36 = property on="RecordsSelection" class="CmbBox"("Text.Text"="") -> ()  [unwired: 2 in, 2 out]
          n37 = call "UpdateDatabaseRemote.vi"("CallType"=enum16{"Initialize", "Save", "Load"}."Initialize") -> ("ExperimentDatesSorted"=w69:string[])  [unwired: 2 in, 2 out]
          n38 = property on="RecordsSelection" class="CmbBox"("Strings[]"=w69) -> ()  [unwired: 2 in, 2 out]
          n39 = local write "Database"(T3 {"ExperimentDate"=timestamp(-9593222400 s since 1904-01-01), "ImplantDate"=timestamp(-9593222400 s since 1904-01-01), "CerebusFolder"="", "Experimenter"="", "PatientNumber"="", "DominantHand"="", "DeviceType"="", "DeviceSerial"="", "DeviceHemisphere"="", "DeviceRegion"="", "TaskType"="", "TaskComments"="", "RecordingComments"="", "GeneralObservations"=""} ("Database")) -> ()
        }
        frame #3 {
          # "Start Cerebus recording"
          n40 = Two Button Dialog(message="Automatically start Central recording?\nIf not, manually start recording now.", 1:"No" ("T button name (\"OK\")"), 2:"Yes" ("T button name (\"OK\")")) -> (T button?=w72:bool)
          n41 = case shown="True" w72 {
            frame False {
              n42 = local write "StopRecording"(FALSE ("StopRecording")) -> ()
            }
            frame True {
              n43 = local read "TaskType"() -> (w94:string)
              n44 = local read "AutoCentraVI"() -> (w83:path)
              n45 = Open Application Reference(10:u16 3362 ("port number or service name (3363)"), 11:"155.101.184.11" ("machine name (\"\":  open local reference)")) -> (0:w86:errorcluster, 3:w88:refnum<vi>)  [unwired: 2 in]
              n46 = local read "SaccadeFolder"() -> (w80:path)
              n47 = Match Pattern(string=w94, regular expression="\\.") -> (before substring=w93:string)  [unwired: 1 in, 3 out]
              n48 = Open VI Reference(type specifier VI Refnum (for type only)=refnum<vi> refnum, application reference (local)=w88, vi path=w83, error in (no error)=w86) -> (vi reference=w84:refnum<vi>, error out=w85:errorcluster)  [unwired: 2 in]
              n49 = Concatenate Strings(w93, "_CerebusConfig.mat" ("string")) -> (w92:string)
              n50 = Build Path(base path=w80, name or relative path=w92) -> (appended path=w81:path)
              n51 = Get Date/Time In Seconds() -> (seconds since 1Jan1904=w82:timestamp)
              n52 = local write "StopRecording"(TRUE ("StopRecording")) -> ()
              n53 = call-by-ref "?"(reference=w84, error in=w85, "ConfigurationFile"=w81, "Mode"=T17."StartRecording") -> ("DataFolder"=w77:string, "Recording?"=w78:bool)  [unwired: 1 in, 3 out]
              n54 = local write "ExperimentDate"(w82) -> ()
              n55 = local write "Recording?"(w78) -> ()
              n56 = local write "CerebusFolder"(w77) -> ()
            }
          }
        }
        frame #4 {
          n57 = disable-structure shown="Disabled" {
            frame Disabled {
              # "Start remote matlab (i.e. Saccade.exe). File should be in C drive of remote computer."
              n58 = local read "RunProgramVI"() -> (w105:path)
              n59 = local read "TaskType"() -> (w101:string)
              n60 = Open Application Reference(10:u16 3362 ("port number or service name (3363)"), 11:"155.101.184.11" ("machine name (\"\":  open local reference)")) -> (0:w108:errorcluster, 3:w110:refnum<vi>)  [unwired: 2 in]
              n61 = Open VI Reference(type specifier VI Refnum (for type only)=refnum<vi> refnum, application reference (local)=w110, vi path=w105, error in (no error)=w108) -> (vi reference=w106:refnum<vi>, error out=w107:errorcluster)  [unwired: 2 in]
              n62 = Search and Replace String(input string=w101, search string=".vi", replace string=".exe" ("replace string (\"\")")) -> (result string=w98:string)  [unwired: 5 in, 3 out]
              n63 = Build Path(base path=path "C:/", name or relative path=w98) -> (appended path=w97:path)
              n64 = call-by-ref "?"(reference=w106, error in=w107, "Program"=w97, "IpAddress"="155.101.184.10", "Mode"=enum16{"Start", "Stop"}."Start") -> ()  [unwired: 3 out]
            }
            frame Enabled {
            }
          }
        }
        frame #5 {
          # "Wait for matlab to start"
          n65 = while {
            stop <- w114 stop-if-true
            n66 = local read "UDPRef"() -> (w115:refnum<k16>)
            n67 = UDP Read(connection ID=w115, timeout ms (25000)=1000) -> (data out=w117:string)  [unwired: 2 in, 4 out]
            n68 = Equal?(x=w117, y="Online") -> (x = y?=w114:bool)
          }
        }
        frame #6 {
          w122 = enum16{"Normal", "Matlab"}."Matlab" ("Type")
          # "Send parameters to matlab: 'LV.ID=SetupInfo;LV.CerebusFolder=20130129-162021;LV.SubjectName=Frik; etc... '"
          n69 = local read "CerebusFolder"() -> (w125:string)
          n70 = call-poly "VariablesToString.vi"("ValueIn"="SetupInfo" ("FieldName"), "FieldName"="ID", "Type"=w122) -> ("StringOut"=w121:string)  [unwired: 4 in]
          n71 = call-poly "VariablesToString.vi"("ValueIn"=w125, "FieldName"="CerebusFolder", "Type"=w122) -> ("StringOut"=w120:string)  [unwired: 4 in]
          n72 = call-poly "VariablesToString.vi"("ValueIn"="Frik", "FieldName"="SubjectName", "Type"=w122) -> ("StringOut"=w119:string)  [unwired: 4 in]
          n73 = Concatenate Strings(w121, w120, w119) -> (w118:string)
          n74 = local read "RemotePort"() -> (w131:u16)
          n75 = local read "RemoteIP"() -> (w130:u32)
          n76 = local read "UDPRef"() -> (w129:refnum<k16>)
          n77 = UDP Write(address=w130, port or service name=w131, connection ID=w129, data in=w118) -> ()  [unwired: 2 in, 2 out]
        }
        frame #7 {
          n78 = Tick Count (ms)() -> (millisecond timer value=w132:u32)
          n79 = local write "ExpStartTime"(w132) -> ()
        }
      }
    }
    frame #1 {
      n80 = node-c288() -> (w134:T24)  [unwired: 2 in]
      n81 = timed-loop {
        timing: w134 -> [_]
        timing-out: [_] -> w133
        i -> [w166]
        stop <- w153 stop-if-true
        w159 = enum16{"In", "Out"}[] [enum."In", enum."In"] items=["In", "Out"] ("y")
        n82 = node-c288() -> (→"Finished Late? [i-1]":bool, w164:i64)  [unwired: 1 in]
        n83 = local read "EyeCalibration"() -> (w146:T15)
        n84 = local read "ExpStartTime"() -> (w181:u32)
        n85 = local read "RecordsSelection"() -> (w143:string)
        n86 = local read "PlotSaccades"() -> (w140:bool)
        n87 = Divide(x=w164, y=i64 1000) -> (x/y=→"LoopPeriod":dbl)
        n88 = call "EyeTracker.vi"("Mode"=enum16{"Initialize", "Run", "Close"}."Run") -> ("EyeXY"=w147:dbl[])
        n89 = feedback #1(w143) -> (w178:string)
        n90 = feedback-in #1(w143) -> ()
        n91 = Get Date/Time In Seconds() -> (seconds since 1Jan1904=w183:timestamp)
        n92 = call "ExperimentTimer.vi"("Experiment Start Time"=w181) -> ("Exp Timer"=w182:u32)
        n93 = call "AdjustEyePos.vi"("EyeCalibration"=w146, "EyeXYIn"=w147) -> ("EyeXYOut"=w144:dbl[])
        n94 = case shown="True" w140 {
          tunnel: [w184 w186] -> w142
          tunnel: [w184 w185] -> w141
          frame False {
            w184 = dbl[][] [] ("initialized array")
          }
          frame True {
            n95 = local read "ElectricArray"() -> (w185:dbl[][])
            n96 = local read "PhoticArray"() -> (w186:dbl[][])
          }
        }
        n97 = local write "ExpTime"(w182) -> ()
        n98 = Equal?(x=w143, y=w178) -> (x = y?=w179:bool)
        n99 = case shown="False" w179 {
          frame False {
            n100 = local read "RecordsSelection"() -> (w1180:string)
            n101 = call "UpdateDatabaseRemote.vi"("RecordsSelection"=w1180, "CallType"=enum16{"Initialize", "Save", "Load"}."Load") -> ("DatabaseOut"=w1181:T3)  [unwired: 1 in, 2 out]
            n102 = local write "Database"(w1181) -> ()
          }
          frame True {
          }
        }
        n103 = local write "Time/Date"(w183) -> ()
        n104 = call "InWindow_Saccade.vi"("EyeCalibration"=w146, "EyeXY"=w144) -> ("EyeStatus"=w145:T5)
        n105 = local write "EyeXY"(w144) -> ()
        n106 = local read "LEDs"() -> (w152:T7)
        n107 = local read "Global Controls"() -> (w162:T11)
        n108 = local read "PhoticBnds"() -> (w137:enum16{"Full Field", "LR Quadrant"})
        n109 = Unbundle By Name(w162) -> ("MonHands"=w161:bool)
        n110 = local write "EyeStatus"(w145) -> ()
        n111 = call "EyePlot.vi"("ElectricArray"=w141, "PhoticArray"=w142, "PhoticBnds"=w137, "LEDs"=w152, "EyeCalibration"=w146, "EyeStatus"=w145, "EyeXY"=w144) -> ("EyeGraph"=w173:cluster{dbl[], dbl[]}[])  [unwired: 4 in]
        n112 = local read "SetElec"() -> (w148:bool)
        n113 = local read "Global Controls"() -> (w172:T11)
        n114 = local write "Eye Graph"(w173) -> ()
        n115 = local read "Elec Indicators"() -> (w136:T8)
        n116 = Unbundle By Name(w145) -> ("Fixation"=w135:enum16{"In", "Out"}, "Photic"=w155:enum16{"In", "Out"}, "Electric"=w139:enum16{"In", "Out"})
        n117 = case shown="True" w161 {
          tunnel: [T18."Both Hands On" ("Hands Status") w195] -> w168
          frame False {
            # "Set Hand Status to On"
          }
          frame True {
            # "Check Hands"
            n118 = call "ReadCapacitanceSwitches.vi"("Mode"=enum32{"Initialize", "Run", "Close"}."Run") -> ("Hands Status"=w195:T18)  [unwired: 2 out]
          }
        }
        n119 = feedback-in #2(w136) -> ()
        n120 = feedback #2() -> (w177:T8)  [unwired: 1 in]
        n121 = case shown="True" w148 {
          frame False {
          }
          frame True {
            n122 = local read "ElectrodeStr"() -> (w191:string)
            n123 = local read "Electrodes"() -> (w190:T9)
            n124 = call "RandomizeElectrodes.vi"("ElectrodeStrIn"=w191, "ElectrodesIn"=w190, "Mode"=enum16{"Set", "Randomize"}."Set") -> ("ElectrodeStrOut"=w192:string, "ElectrodesOut"=w189:T9)  [unwired: 1 in]
            n125 = local write "SetElec"(FALSE ("SetElec")) -> ()
            n126 = local write "Electrodes"(w189) -> ()
            n127 = local write "ElectrodeStr"(w192) -> ()
          }
        }
        n128 = Build Array(w135, w155) -> (w154:enum16{"In", "Out"}[])
        n129 = Unbundle By Name(w172) -> ("TrackEyes"=w171:bool)
        n130 = Equal?(x=w136, y=w177) -> (x = y?=w176:T27)
        n131 = Equal?(x=w154, y=w159) -> (x = y?=w158:bool[])
        n132 = Cluster To Array(cluster=w176) -> (array=w175:bool[])
        n133 = Or Array Elements(Boolean array=w158) -> (logical OR=w160:bool)
        n134 = And Array Elements(Boolean array=w175) -> (logical AND=w174:bool)
        n135 = case shown="\"Both Hands On\"" w168 {
          frame "Both Hands Off", Default {
            n136 = local read "LEDs"() -> (w203:T7)
            n137 = Bundle By Name(cluster=w203, "HandsReady"=FALSE ("LED Hands Ready"), "RightHand"=FALSE ("LED Right Hand"), "LeftHand"=FALSE ("LED Left Hand")) -> (w202:T7)
            n138 = local write "LEDs"(w202) -> ()
          }
          frame "Both Hands On" {
            n139 = local read "LEDs"() -> (w208:T7)
            n140 = Bundle By Name(cluster=w208, "HandsReady"=TRUE ("LED Hands Ready"), "RightHand"=TRUE ("LED Right Hand"), "LeftHand"=TRUE ("LED Left Hand")) -> (w207:T7)
            n141 = local write "LEDs"(w207) -> ()
          }
          frame "Left Hand Off" {
            n142 = local read "LEDs"() -> (w213:T7)
            n143 = Bundle By Name(cluster=w213, "HandsReady"=FALSE ("LED Hands Ready"), "RightHand"=TRUE ("LED Right Hand"), "LeftHand"=FALSE ("LED Left Hand")) -> (w212:T7)
            n144 = local write "LEDs"(w212) -> ()
          }
          frame "Right Hand Off" {
            n145 = local read "LEDs"() -> (w218:T7)
            n146 = Bundle By Name(cluster=w218, "HandsReady"=FALSE ("LED Hands Ready"), "RightHand"=FALSE ("LED Right Hand"), "LeftHand"=TRUE ("LED Left Hand")) -> (w217:T7)
            n147 = local write "LEDs"(w217) -> ()
          }
        }
        n148 = case shown="True" w171 {
          tunnel: w135 -> [_ w225]
          tunnel: w155 -> [_ w224]
          tunnel: [w222 w225] -> w157
          tunnel: [w222 w224] -> w156
          tunnel: w139 -> [_ w223]
          tunnel: [w222 w223] -> w138
          frame False {
            w222 = enum16{"In", "Out"}."In" ("Status")
            # "Set In Window Vals to In"
          }
          frame True {
            # "Pass In Window Booleans"
          }
        }
        n149 = case shown="False" w160 {
          frame False {
            n150 = local read "LEDs"() -> (w197:T7)
            n151 = Bundle By Name(cluster=w197, "InRange"=FALSE ("LED Fixation")) -> (w196:T7)
            n152 = local write "LEDs"(w196) -> ()
          }
          frame True {
            n153 = local read "LEDs"() -> (w200:T7)
            n154 = Bundle By Name(cluster=w200, "InRange"=TRUE ("LED Fixation")) -> (w199:T7)
            n155 = local write "LEDs"(w199) -> ()
          }
        }
        n156 = local read "TrialStatus"() -> (w167:T2)
        n157 = Bundle By Name(cluster=w167, "HandsStatus"=w168) -> (w169:T2)
        n158 = case shown="False" w174 {
          tunnel: w136 -> [_ _]
          frame False {
            n159 = local read "Elec Indicators"() -> (w1177:T8)
            n160 = call "StimCalc.vi"("Elec Indicators In"=w1177) -> ("Damage Plot"=w1178:cluster{"Y":dbl[], "Y":dbl[]}[], "Elec Indicators Out"=w1176:T8)  [unwired: 1 in]
            n161 = local write "Elec Indicators"(w1176) -> ()
            n162 = local write "Damage Plot"(w1178) -> ()
          }
          frame True {
          }
        }
        n163 = Unbundle By Name(w167) -> ("TrialState"=w170:T21, "InitializeState"=w149:T22, "FinalizeState"=w150:T22)
        n164 = local write "TrialStatus"(w169) -> ()
        n165 = case shown="\"Initialize\", Default" w170 {
          tunnel: w168 -> [_ w441 w480 _]
          tunnel: w157 -> [_ w431 w479 _]
          tunnel: w156 -> [_ _ w478 _]
          tunnel: [_ _ _ w650] -> w153
          tunnel: w150 -> [_ _ _ w649]
          tunnel: w149 -> [w226 _ _ _]
          tunnel: w138 -> [_ _ w477 _]
          frame "Initialize", Default {
            n166 = case shown="\"4\"" w226 {
              frame "0" {
                # "Determining StimType (Electric/Photic)"
                n167 = local read "StimButton"() -> (w229:bool)
                n168 = local read "TrialStatus"() -> (w228:T2)
                n169 = case shown="True" w229 {
                  tunnel: w228 -> [w232 w239]
                  tunnel: [w234 w238] -> w227
                  frame False {
                    w230 = enum32{"---", "Photic", "Electric"}."Photic" ("StimType")
                    n170 = Unbundle By Name(w232) -> ("InitializeState"=w233:T22)
                    n171 = Increment(x=w233) -> (x+1=w231:T22)
                    n172 = Bundle By Name(cluster=w232, "InitializeState"=w231, "StimType"=w230) -> (w234:T2)
                    n173 = local write "StimTypeBigIndicator"(w230) -> ()
                  }
                  frame True {
                    n174 = local read "StimSwitchSettings"() -> (w243:T6)
                    n175 = Unbundle By Name(w243) -> ("ElecStimMode"=w242:enum16{"Continuous", "Manual"}, "ElecPerc"=w241:dbl)
                    n176 = Unbundle By Name(w239) -> ("InitializeState"=w237:T22, "StimType"=w240:enum32{"---", "Photic", "Electric"})
                    n177 = case shown="\"Continuous\", Default" w242 {
                      tunnel: [w246 enum32{"---", "Photic", "Electric"}."Electric" ("StimType")] -> w235
                      tunnel: w241 -> [w245 _]
                      tunnel: w240 -> [w244 _]
                      frame "Continuous", Default {
                        n178 = case shown="\"Photic\", Default" w244 {
                          tunnel: [w250 w256] -> w246
                          tunnel: w245 -> [w247 w255]
                          frame "Photic", Default {
                            n179 = Random Number (0-1)() -> (number: 0 to 1=w248:dbl)
                            n180 = Less?(x=w248, y=w247) -> (x < y?=w249:bool)
                            n181 = case shown="True" w249 {
                              tunnel: [enum32{"---", "Photic", "Electric"}."Photic" ("StimType") enum32{"---", "Photic", "Electric"}."Electric" ("StimType")] -> w250
                              frame False {
                              }
                              frame True {
                              }
                            }
                          }
                          frame "Electric" {
                            n182 = Equal?(x=w255, y=1.0) -> (x = y?=w253:bool)
                            n183 = case shown="False" w253 {
                              tunnel: [enum32{"---", "Photic", "Electric"}."Photic" ("StimType") enum32{"---", "Photic", "Electric"}."Electric" ("StimType")] -> w256
                              frame False {
                              }
                              frame True {
                              }
                            }
                          }
                        }
                      }
                      frame "Manual" {
                      }
                    }
                    n184 = Increment(x=w237) -> (x+1=w236:T22)
                    n185 = Bundle By Name(cluster=w239, "InitializeState"=w236, "StimType"=w235) -> (w238:T2)
                    n186 = local write "StimTypeBigIndicator"(w235) -> ()
                  }
                }
                n187 = local write "TrialStatus"(w227) -> ()
              }
              frame "1" {
                w270 = enum16{"Normal", "Matlab"}."Matlab" ("Type")
                # "Draw Fixation"
                n188 = local read "PhoticStimSettings"() -> (w263:T13)
                n189 = local read "EyeCalibration"() -> (w278:T15)
                n190 = local read "TrialStatus"() -> (w280:T2)
                n191 = Unbundle By Name(w263) -> ("BGnd"=w262:dbl)
                n192 = Unbundle By Name(w278) -> ("Fix.X"=w266:dbl, "Fix.Y"=w265:dbl)
                n193 = Unbundle By Name(w280) -> ("InitializeState"=w279:T22)
                n194 = Increment(x=w279) -> (x+1=w281:T22)
                n195 = call-poly "VariablesToString.vi"("ValueIn"="DrawFix" ("FieldName"), "FieldName"="ID", "Type"=w270) -> ("StringOut"=w269:string)  [unwired: 4 in]
                n196 = call-poly "VariablesToString.vi"("ValueIn"=w266, "FieldName"="FixX", "Type"=w270) -> ("StringOut"=w268:string)  [unwired: 4 in]
                n197 = call-poly "VariablesToString.vi"("ValueIn"=w265, "FieldName"="FixY", "Type"=w270) -> ("StringOut"=w267:string)  [unwired: 4 in]
                n198 = call-poly "VariablesToString.vi"("ValueIn"=w262, "FieldName"="LV.BGnd") -> ("StringOut"=w260:string)  [unwired: 5 in]
                n199 = Bundle By Name(cluster=w280, "InitializeState"=w281) -> (w282:T2)
                n200 = Concatenate Strings(w269, w268, w267, w260) -> (w264:string)
                n201 = local read "RemotePort"() -> (w277:u16)
                n202 = local read "RemoteIP"() -> (w276:u32)
                n203 = local read "UDPRef"() -> (w275:refnum<k16>)
                n204 = local write "TrialStatus"(w282) -> ()
                n205 = UDP Write(address=w276, port or service name=w277, connection ID=w275, data in=w264) -> ()  [unwired: 2 in, 2 out]
              }
              frame "2" {
                # "Randomize parameters"
                n206 = local read "TrialStatus"() -> (w286:T2)
                n207 = Unbundle By Name(w286) -> ("InitializeState"=w285:T22, "StimType"=w284:enum32{"---", "Photic", "Electric"}, "Outcome"=w283:enum32{"---", "Success", "Abort"})
                n208 = Increment(x=w285) -> (x+1=w287:T22)
                n209 = Bundle By Name(cluster=w286, "InitializeState"=w287) -> (w288:T2)
                n210 = case shown="\"Electric\"" w284 {
                  tunnel: w283 -> [w289 _]
                  frame "Photic", Default {
                    n211 = local read "RandPhotic"() -> (w290:bool)
                    n212 = case shown="True" w290 {
                      tunnel: w289 -> [_ w292]
                      frame False {
                        n213 = local write "RandFlag"(FALSE ("RandFlag")) -> ()
                      }
                      frame True {
                        n214 = case shown="\"Abort\"" w292 {
                          frame "Abort" {
                            n215 = local read "AbortCount"() -> (w295:u64)
                            n216 = Less?(x=w295, y=u64 4) -> (x < y?=w293:bool)
                            n217 = case shown="False" w293 {
                              frame False {
                                n218 = local write "AbortCount"(u64 0 ("AbortCount")) -> ()
                                n219 = local write "RandFlag"(TRUE ("RandFlag")) -> ()
                              }
                              frame True {
                                n220 = local read "AbortCount"() -> (w300:u64)
                                n221 = local write "RandFlag"(FALSE ("RandFlag")) -> ()
                                n222 = Increment(x=w300) -> (x+1=w299:u64)
                                n223 = local write "AbortCount"(w299) -> ()
                              }
                            }
                          }
                          frame "Success", Default {
                            n224 = local write "AbortCount"(u64 0 ("AbortCount")) -> ()
                            n225 = local write "RandFlag"(TRUE ("RandFlag")) -> ()
                          }
                        }
                      }
                    }
                  }
                  frame "Electric" {
                    n226 = local read "ElectrodeStr"() -> (w306:string)
                    n227 = local read "Electrodes"() -> (w305:T9)
                    n228 = call "RandomizeElectrodes.vi"("ElectrodeStrIn"=w306, "ElectrodesIn"=w305, "Mode"=enum16{"Set", "Randomize"}."Randomize") -> ("ElectrodeStrOut"=w307:string, "ElectrodesOut"=w304:T9)  [unwired: 1 in]
                    n229 = local write "Electrodes"(w304) -> ()
                    n230 = local write "ElectrodeStr"(w307) -> ()
                  }
                }
                n231 = local write "TrialStatus"(w288) -> ()
              }
              frame "3" {
                # "Update stimulus settings, reset array"
                n232 = local read "RandPhotic"() -> (w312:bool)
                n233 = local read "ArrayReset"() -> (w317:bool)
                n234 = local read "TrialStatus"() -> (w314:T2)
                n235 = case shown="True" w317 {
                  frame False {
                  }
                  frame True {
                    n236 = for {
                      N: 100 -> [_]
                      tunnel: [0] -> w359 mode=indexing
                    }
                    n237 = Array To Cluster(array=w359) -> (cluster=w358:T28)
                    n238 = local write "Electrodes"(w358) -> ()
                    n239 = local write "ArrayReset"(FALSE ("Array Reset")) -> ()
                  }
                }
                n240 = local read "PhoticStimSettings"() -> (w308:T13)
                n241 = case shown="False" w312 {
                  tunnel: [w319 w328] -> w310
                  tunnel: [w318 w327] -> w309
                  tunnel: w308 -> [_ w326]
                  frame False {
                    n242 = local read "PhoticStimPresets"() -> (w325:T4)
                    n243 = To Unsigned Long Integer(number=w325) -> (unsigned 32bit integer=w324:u32)
                    n244 = call "GenPhoticPos.vi"("PhoticBnds"=enum16{"Full Field", "LR Quadrant"}."Full Field") -> ("Y"=w322:dbl[], "X"=w323:dbl[])  [unwired: 3 in, 2 out]
                    n245 = Decrement(x=w324) -> (x-1=w321:u32)
                    n246 = Index Array(array=w323, index=w321) -> (element=w319:dbl)
                    n247 = Index Array(array=w322, index=w321) -> (element=w318:dbl)
                  }
                  frame True {
                    n248 = local read "RandFlag"() -> (w329:bool)
                    n249 = case shown="True" w329 {
                      tunnel: [w332 w334] -> w328
                      tunnel: [w331 w333] -> w327
                      tunnel: w326 -> [w330 _]
                      frame False {
                        n250 = Unbundle By Name(w330) -> ("StimX"=w332:dbl, "StimY"=w331:dbl)
                      }
                      frame True {
                        n251 = local read "PhoticBnds"() -> (w335:enum16{"Full Field", "LR Quadrant"})
                        n252 = case shown="\"LR Quadrant\"" w335 {
                          tunnel: w335 -> [w342 w353]
                          tunnel: [w341 w350] -> w334
                          tunnel: [w340 w349] -> w333
                          frame "Full Field", Default {
                            n253 = Random Number (0-1)() -> (number: 0 to 1=w346:dbl)
                            n254 = Multiply(x=w346, y=16.0) -> (x*y=w343:dbl)
                            n255 = call "GenPhoticPos.vi"("PhoticBnds"=w342) -> ("Y"=w338:dbl[], "X"=w339:dbl[])  [unwired: 3 in, 2 out]
                            n256 = Add(x=w343, y=9.0) -> (x+y=w344:dbl)
                            n257 = Round Toward -Infinity(1:w344) -> (0:w337:dbl)
                            n258 = Decrement(x=w337) -> (x-1=w336:dbl)
                            n259 = Index Array(array=w339, index=w336) -> (element=w341:dbl)
                            n260 = Index Array(array=w338, index=w336) -> (element=w340:dbl)
                          }
                          frame "LR Quadrant" {
                            n261 = Random Number (0-1)() -> (number: 0 to 1=w356:dbl)
                            n262 = call "GenPhoticPos.vi"("PhoticBnds"=w353) -> ("Y"=w351:dbl[], "X"=w352:dbl[])  [unwired: 3 in, 2 out]
                            n263 = Multiply(x=w356, y=11.0) -> (x*y=w354:dbl)
                            n264 = Round Toward -Infinity(1:w354) -> (0:w348:dbl)
                            n265 = Index Array(array=w352, index=w348) -> (element=w350:dbl)
                            n266 = Index Array(array=w351, index=w348) -> (element=w349:dbl)
                          }
                        }
                      }
                    }
                  }
                }
                n267 = Unbundle By Name(w314) -> ("InitializeState"=w313:T22)
                n268 = Increment(x=w313) -> (x+1=w315:T22)
                n269 = Bundle By Name(cluster=w314, "InitializeState"=w315) -> (w316:T2)
                n270 = local write "TrialStatus"(w316) -> ()
                n271 = Bundle By Name(cluster=w308, "StimX"=w310, "StimY"=w309) -> (w311:T13)
                n272 = local write "PhoticStimSettings"(w311) -> ()
              }
              frame "4" {
                # "Draw EStim or PStim in Matlab"
                n273 = local read "TrialStatus"() -> (w372:T2)
                n274 = local read "PhoticStimSettings"() -> (w369:T13)
                n275 = local read "ElecStimSettings"() -> (w367:T1)
                n276 = local read "TrialStatus"() -> (w366:T2)
                n277 = local read "Electrodes"() -> (w370:T9)
                n278 = Unbundle By Name(w372) -> ("InitializeState"=w371:T22)
                n279 = call "MatlabStimCom.vi"("TrialStatus"=w366, "PhoticStimSettings"=w369, "ElecStimSettings"=w367, "Electrodes"=w370) -> ("MATLABCom"=w362:string, "Current Electrode"=w368:i32)  [unwired: 1 in]
                n280 = Increment(x=w371) -> (x+1=w373:T22)
                n281 = local write "Current Electrode"(w368) -> ()
                n282 = Bundle By Name(cluster=w372, "InitializeState"=w373) -> (w374:T2)
                n283 = local write "MATLABCom"(w362) -> ()
                n284 = local write "TrialStatus"(w374) -> ()
                n285 = local read "RemotePort"() -> (w365:u16)
                n286 = local read "RemoteIP"() -> (w364:u32)
                n287 = local read "UDPRef"() -> (w363:refnum<k16>)
                n288 = UDP Write(address=w364, port or service name=w365, connection ID=w363, data in=w362) -> ()  [unwired: 2 in, 2 out]
              }
              frame "5" {
                # "Update stimulus window based on location of stimulus"
                n289 = local read "TrialStatus"() -> (w380:T2)
                n290 = Unbundle By Name(w380) -> ("StimType"=w379:enum32{"---", "Photic", "Electric"})
                n291 = case shown="\"Photic\", Default" w379 {
                  frame "Photic", Default {
                    n292 = local read "PhoticStimSettings"() -> (w385:T13)
                    n293 = Unbundle By Name(w385) -> ("StimX"=w382:dbl, "StimY"=w381:dbl)
                    n294 = local read "EyeCalibration"() -> (w384:T15)
                    n295 = Bundle By Name(cluster=w384, "Photic.X"=w382, "Photic.Y"=w381) -> (w383:T15)
                    n296 = local write "EyeCalibration"(w383) -> ()
                  }
                  frame "Electric" {
                  }
                }
                n297 = local read "TrialStatus"() -> (w376:T2)
                n298 = Unbundle By Name(w376) -> ("InitializeState"=w375:T22)
                n299 = Increment(x=w375) -> (x+1=w377:T22)
                n300 = Bundle By Name(cluster=w376, "InitializeState"=w377) -> (w378:T2)
                n301 = local write "TrialStatus"(w378) -> ()
              }
              frame "6" {
                n302 = local read "TrialStatus"() -> (w387:T2)
                n303 = Unbundle By Name(w387) -> ("InitializeState"=w386:T22)
                n304 = Increment(x=w386) -> (x+1=w388:T22)
                n305 = Bundle By Name(cluster=w387, "InitializeState"=w388) -> (w389:T2)
                n306 = local write "TrialStatus"(w389) -> ()
              }
              frame "7" {
                n307 = local read "TrialStatus"() -> (w391:T2)
                n308 = Unbundle By Name(w391) -> ("InitializeState"=w390:T22)
                n309 = Increment(x=w390) -> (x+1=w392:T22)
                n310 = Bundle By Name(cluster=w391, "InitializeState"=w392) -> (w393:T2)
                n311 = local write "TrialStatus"(w393) -> ()
              }
              frame "8" {
                n312 = local read "TrialStatus"() -> (w395:T2)
                n313 = Unbundle By Name(w395) -> ("InitializeState"=w394:T22)
                n314 = Increment(x=w394) -> (x+1=w396:T22)
                n315 = Bundle By Name(cluster=w395, "InitializeState"=w396) -> (w397:T2)
                n316 = local write "TrialStatus"(w397) -> ()
              }
              frame "9" {
                n317 = local read "TrialStatus"() -> (w399:T2)
                n318 = Unbundle By Name(w399) -> ("InitializeState"=w398:T22)
                n319 = Increment(x=w398) -> (x+1=w400:T22)
                n320 = Bundle By Name(cluster=w399, "InitializeState"=w400) -> (w401:T2)
                n321 = local write "TrialStatus"(w401) -> ()
              }
              frame "10" {
                # "Turn Fixation On"
                n322 = local read "LoopCount"() -> (w404:u64)
                n323 = call "RunOnce.vi"("Instance"=0, "Mode"=enum16{"Reset", "Run"}."Reset") -> ()  [unwired: 1 out]
                n324 = call "LoopComp.vi"("LoopCount"=w404, "Instance"=0, "Mode"=enum16{"Reset", "Run"}."Reset") -> ()  [unwired: 3 in, 2 out]
                n325 = local read "TrialStatus"() -> (w422:T2)
                n326 = Bundle By Name(cluster=w422, "TrialState"=T21."Acquire Fixation", "InitializeState"=T22."0", "FinalizeState"=T22."0", "Outcome"=enum32{"---", "Success", "Abort"}."---", "AbortLocation"=T20."---", "AbortReason"=T19."---") -> (w423:T2)
                n327 = local write "SAFlag"(FALSE ("SAFlag")) -> ()
                n328 = local write "WfFlag"(FALSE ("SAFlag")) -> ()
                n329 = local write "TrialStatus"(w423) -> ()
                n330 = local read "RemotePort"() -> (w409:u16)
                n331 = local read "RemoteIP"() -> (w410:u32)
                n332 = local read "UDPRef"() -> (w411:refnum<k16>)
                n333 = UDP Write(address=w410, port or service name=w409, connection ID=w411, data in="LV.ID='FixOn';") -> ()  [unwired: 2 in, 2 out]
                n334 = call-poly <vilib>:"DAQmx Write.vi"("task/channels in"=refnum<k21> "Juice", "data"=0.0) -> ()  [unwired: 11 in, 3 out]
                n335 = local read "LEDs"() -> (w416:T7)
                n336 = Bundle By Name(cluster=w416, "Fixation"=TRUE ("LED Fixation")) -> (w415:T7)
                n337 = local write "LEDs"(w415) -> ()
              }
            }
          }
          frame "Acquire Fixation" {
            # "Establish Hands Ready and Eyes in Fixation"
            n338 = local read "Timers"() -> (w438:T12)
            n339 = local read "LoopPeriod"() -> (w432:u64)
            n340 = local read "LoopCount"() -> (w426:u64)
            n341 = Unbundle By Name(w438) -> ("ST.AFD"=w436:u64, "RT.AFD"=w435:u64)
            n342 = call "LoopComp.vi"("RandTime"=w435, "LoopPeriod"=w432, "SetTime"=w436, "LoopCount"=w426, "Instance"=0, "Mode"=enum16{"Reset", "Run"}."Run") -> ("ActualTime"=w439:u64, "Outcome"=w440:enum16{"TimeIn", "TimeOut"})
            n343 = Bundle By Name(cluster=w438, "AT.AFD"=w439) -> (w437:T12)
            n344 = local write "Timers"(w437) -> ()
            n345 = case shown="\"Both Hands On\"" w441 {
              tunnel: w431 -> [_ w451]
              tunnel: w440 -> [_ w452]
              frame "Both Hands Off", Default {
                n346 = local read "LoopCount"() -> (w448:u64)
                n347 = call "LoopComp.vi"("LoopCount"=w448, "Instance"=0, "Mode"=enum16{"Reset", "Run"}."Reset") -> ()  [unwired: 3 in, 2 out]
              }
              frame "Both Hands On" {
                n348 = case shown="\"In\"" w451 {
                  tunnel: w452 -> [w453 _]
                  frame "In" {
                    # "Eyes In"
                    n349 = case shown="\"TimeOut\"" w453 {
                      frame "TimeIn", Default {
                        # "Counting Up"
                      }
                      frame "TimeOut" {
                        w454 = enum16{"Reset", "Run"}."Reset" ("Mode")
                        w455 = enum16{"Reset", "Run"}."Reset" ("Mode")
                        # "Move to Next State"
                        n350 = local read "LoopCount"() -> (w456:u64)
                        n351 = local read "TrialStatus"() -> (w472:T2)
                        n352 = call "LoopComp.vi"("LoopCount"=w456, "Instance"=0, "Mode"=w455) -> ()  [unwired: 3 in, 2 out]
                        n353 = call "LoopComp.vi"("LoopCount"=w456, "Instance"=1, "Mode"=w455) -> ()  [unwired: 3 in, 2 out]
                        n354 = call "LoopComp.vi"("LoopCount"=w456, "Instance"=2, "Mode"=w455) -> ()  [unwired: 3 in, 2 out]
                        n355 = call "LoopComp.vi"("LoopCount"=w456, "Instance"=3, "Mode"=w455) -> ()  [unwired: 3 in, 2 out]
                        n356 = call "LoopComp.vi"("LoopCount"=w456, "Instance"=4, "Mode"=w455) -> ()  [unwired: 3 in, 2 out]
                        n357 = call "SendCerebus8.vi"("String"="FixationAcquired" ("ASCII Data"), "Mode"=T16."String") -> ()  [unwired: 3 in]
                        n358 = Bundle By Name(cluster=w472, "TrialState"=T21."Visual Stimuli") -> (w473:T2)
                        n359 = local write "TrialStatus"(w473) -> ()
                        n360 = local read "LEDs"() -> (w468:T7)
                        n361 = Bundle By Name(cluster=w468, "TaskInProgress"=TRUE ("LED Fixation")) -> (w467:T7)
                        n362 = local write "LEDs"(w467) -> ()
                        n363 = call "RunOnce.vi"("Instance"=0, "Mode"=w454) -> ()  [unwired: 1 out]
                        n364 = call "RunOnce.vi"("Instance"=1, "Mode"=w454) -> ()  [unwired: 1 out]
                        n365 = call "RunOnce.vi"("Instance"=2, "Mode"=w454) -> ()  [unwired: 1 out]
                        n366 = call "RunOnce.vi"("Instance"=3, "Mode"=w454) -> ()  [unwired: 1 out]
                      }
                    }
                  }
                  frame "Out", Default {
                    # "Eyes Out"
                    n367 = local read "LoopCount"() -> (w474:u64)
                    n368 = call "LoopComp.vi"("LoopCount"=w474, "Instance"=0, "Mode"=enum16{"Reset", "Run"}."Reset") -> ()  [unwired: 3 in, 2 out]
                  }
                }
              }
            }
            n369 = local read "Global Controls"() -> (w430:T11)
            n370 = Unbundle By Name(w430) -> ("Stop"=w429:bool, "Pause"=w428:bool)
            n371 = Or(x=w429, y=w428) -> (x .or. y?=w427:bool)
            n372 = case shown="False" w427 {
              frame False {
              }
              frame True {
                n373 = local read "TrialStatus"() -> (w444:T2)
                n374 = Bundle By Name(cluster=w444, "TrialState"=T21."Finalize", "Outcome"=enum32{"---", "Success", "Abort"}."---", "AbortLocation"=T20."---", "AbortReason"=T19."---") -> (w447:T2)
                n375 = local write "TrialStatus"(w447) -> ()
              }
            }
          }
          frame "Visual Stimuli" {
            n376 = case shown="\"Both Hands On\"" w480 {
              tunnel: w479 -> [_ w495]
              tunnel: w478 -> [_ w494]
              tunnel: w477 -> [_ w493]
              frame "Both Hands Off", Default {
                n377 = local read "TrialStatus"() -> (w485:T2)
                n378 = Bundle By Name(cluster=w485, "TrialState"=T21."Finalize", "Outcome"=enum32{"---", "Success", "Abort"}."Abort", "AbortLocation"=T20."Visual Stimuli", "AbortReason"=T19."Removed Hands") -> (w486:T2)
                n379 = local write "TrialStatus"(w486) -> ()
              }
              frame "Both Hands On" {
                # "Hold Fixation Timer"
                n380 = local read "Timers"() -> (w498:T12)
                n381 = local read "Timers"() -> (w487:T12)
                n382 = local read "LoopPeriod"() -> (w503:u64)
                n383 = local read "LoopCount"() -> (w490:u64)
                n384 = local read "LoopPeriod"() -> (w507:u64)
                n385 = local read "LoopCount"() -> (w491:u64)
                n386 = Unbundle By Name(w498) -> ("ST.HF"=w500:u64, "RT.HF"=w504:u64)
                n387 = Unbundle By Name(w487) -> ("ST.SD"=w509:u64, "RT.SD"=w505:u64)
                n388 = call "LoopComp.vi"("RandTime"=w504, "LoopPeriod"=w503, "SetTime"=w500, "LoopCount"=w490, "Instance"=1, "Mode"=enum16{"Reset", "Run"}."Run") -> ("ActualTime"=w497:u64, "Outcome"=w496:enum16{"TimeIn", "TimeOut"})
                n389 = Bundle By Name(cluster=w498, "AT.HF"=w497) -> (w499:T12)
                n390 = local write "Timers"(w499) -> ()
                n391 = call "LoopComp.vi"("RandTime"=w505, "LoopPeriod"=w507, "SetTime"=w509, "LoopCount"=w491, "Instance"=0, "Mode"=enum16{"Reset", "Run"}."Run") -> ("ActualTime"=w489:u64, "Outcome"=w506:enum16{"TimeIn", "TimeOut"})
                n392 = Bundle By Name(cluster=w487, "AT.SD"=w489) -> (w488:T12)
                n393 = local write "Timers"(w488) -> ()
                n394 = case shown="\"TimeOut\"" w496 {
                  tunnel: w495 -> [w510 _]
                  tunnel: w494 -> [_ w531]
                  tunnel: w493 -> [_ w529]
                  frame "TimeIn", Default {
                    n395 = case shown="\"Out\"" w510 {
                      frame "In", Default {
                        # "Must Hold Fixation While PStim is Applied"
                        n396 = local read "LoopCount"() -> (w514:u64)
                        n397 = local read "LoopCount"() -> (w513:u64)
                        n398 = call "LoopComp.vi"("LoopCount"=w514, "Instance"=2, "Mode"=enum16{"Reset", "Run"}."Reset") -> ()  [unwired: 3 in, 2 out]
                        n399 = call "LoopComp.vi"("LoopCount"=w513, "Instance"=3, "Mode"=enum16{"Reset", "Run"}."Reset") -> ()  [unwired: 3 in, 2 out]
                      }
                      frame "Out" {
                        # "Lost Fixation = Abort"
                        n400 = local read "TrialStatus"() -> (w521:T2)
                        n401 = Bundle By Name(cluster=w521, "TrialState"=T21."Finalize", "Outcome"=enum32{"---", "Success", "Abort"}."Abort", "AbortLocation"=T20."Hold Fixation", "AbortReason"=T19."Looked Away") -> (w522:T2)
                        n402 = local write "TrialStatus"(w522) -> ()
                      }
                    }
                  }
                  frame "TimeOut" {
                    # "Held Fixation Throughout Stim - Now Check Saccade Location"
                    n403 = local read "TrialStatus"() -> (w533:T2)
                    n404 = local read "Timers"() -> (w539:T12)
                    n405 = local read "LoopCount"() -> (w524:u64)
                    n406 = call "RunOnce.vi"("Instance"=2, "Mode"=enum16{"Reset", "Run"}."Run") -> ("State"=w526:enum16{"RunOnce", "Finished"})
                    n407 = local read "LoopPeriod"() -> (w535:u64)
                    n408 = Unbundle By Name(w533) -> ("StimType"=w532:enum32{"---", "Photic", "Electric"})
                    n409 = Unbundle By Name(w539) -> ("ST.HS"=w537:u64, "RT.HS"=w534:u64)
                    n410 = case shown="\"RunOnce\", Default" w526 {
                      frame "RunOnce", Default {
                        # "Turn Off Fixation"
                        n411 = local read "LEDs"() -> (w546:T7)
                        n412 = Bundle By Name(cluster=w546, "Fixation"=FALSE ("LED Fixation")) -> (w545:T7)
                        n413 = local write "LEDs"(w545) -> ()
                        n414 = local read "RemoteIP"() -> (w544:u32)
                        n415 = local read "RemotePort"() -> (w543:u16)
                        n416 = local read "UDPRef"() -> (w549:refnum<k16>)
                        n417 = UDP Write(address=w544, port or service name=w543, connection ID=w549, data in="LV.ID='FixOff';") -> ()  [unwired: 2 in, 2 out]
                      }
                      frame "Finished" {
                      }
                    }
                    n418 = case shown="\"Electric\"" w532 {
                      tunnel: w531 -> [w541 _]
                      tunnel: [w541 w542] -> w530
                      tunnel: w529 -> [_ w542]
                      frame "Photic", Default {
                        # "Pass Eyes In Window Bool"
                      }
                      frame "Electric" {
                        # "Pass Eyes In Window Bool"
                      }
                    }
                    n419 = call "LoopComp.vi"("RandTime"=w534, "LoopPeriod"=w535, "SetTime"=w537, "LoopCount"=w524, "Instance"=2, "Mode"=enum16{"Reset", "Run"}."Run") -> ("ActualTime"=w540:u64, "Outcome"=w523:enum16{"TimeIn", "TimeOut"})
                    n420 = Bundle By Name(cluster=w539, "AT.HS"=w540) -> (w538:T12)
                    n421 = local write "Timers"(w538) -> ()
                    n422 = case shown="\"TimeIn\", Default" w523 {
                      tunnel: w530 -> [w550 _]
                      frame "TimeIn", Default {
                        n423 = case shown="\"Out\"" w550 {
                          frame "In", Default {
                            # "Saccade Overshoot Timer"
                            n424 = local read "LoopPeriod"() -> (w558:u64)
                            n425 = local read "LoopCount"() -> (w554:u64)
                            n426 = local read "LoopCount"() -> (w551:u64)
                            n427 = call "LoopComp.vi"("LoopPeriod"=w558, "SetTime"=u64 50, "LoopCount"=w554, "Instance"=4, "Mode"=enum16{"Reset", "Run"}."Run") -> ("Outcome"=w557:enum16{"TimeIn", "TimeOut"})  [unwired: 1 in, 1 out]
                            n428 = case shown="\"TimeIn\", Default" w557 {
                              frame "TimeIn", Default {
                                # "Wait During Overshoot Time"
                              }
                              frame "TimeOut" {
                                # "Send StimAcq to Cerebus"
                                n429 = call "RunOnce.vi"("Instance"=3, "Mode"=enum16{"Reset", "Run"}."Run") -> ("State"=w560:enum16{"RunOnce", "Finished"})
                                n430 = case shown="\"RunOnce\", Default" w560 {
                                frame "RunOnce", Default {
                                n431 = local write "SAFlag"(TRUE ("SAFlag")) -> ()
                                n432 = call "SendCerebus8.vi"("String"="StimAcquired" ("ASCII Data"), "Mode"=T16."String") -> ()  [unwired: 3 in]
                                }
                                frame "Finished" {
                                }
                                }
                              }
                            }
                            n433 = call "LoopComp.vi"("LoopCount"=w551, "Instance"=3, "Mode"=enum16{"Reset", "Run"}."Reset") -> ()  [unwired: 3 in, 2 out]
                          }
                          frame "Out" {
                            n434 = local read "SAFlag"() -> (w566:bool)
                            n435 = case shown="False" w566 {
                              frame False {
                                w572 = enum16{"Reset", "Run"}."Reset" ("Mode")
                                # "If Out for too long, Abort Trial"
                                n436 = local read "LoopCount"() -> (w573:u64)
                                n437 = local read "LoopPeriod"() -> (w569:u64)
                                n438 = local read "LoopCount"() -> (w567:u64)
                                n439 = local read "Timers"() -> (w576:T12)
                                n440 = Unbundle By Name(w576) -> ("ST.AS"=w579:u64, "RT.AS"=w577:u64)
                                n441 = call "LoopComp.vi"("LoopCount"=w573, "Instance"=2, "Mode"=w572) -> ()  [unwired: 3 in, 2 out]
                                n442 = call "LoopComp.vi"("LoopCount"=w573, "Instance"=4, "Mode"=w572) -> ()  [unwired: 3 in, 2 out]
                                n443 = call "LoopComp.vi"("RandTime"=w577, "LoopPeriod"=w569, "SetTime"=w579, "LoopCount"=w567, "Instance"=3, "Mode"=enum16{"Reset", "Run"}."Run") -> ("ActualTime"=w575:u64, "Outcome"=w578:enum16{"TimeIn", "TimeOut"})
                                n444 = Bundle By Name(cluster=w576, "AT.AS"=w575) -> (w574:T12)
                                n445 = local write "Timers"(w574) -> ()
                                n446 = case shown="\"TimeOut\"" w578 {
                                frame "TimeIn", Default {
                                }
                                frame "TimeOut" {
                                n447 = local read "TrialStatus"() -> (w585:T2)
                                n448 = Bundle By Name(cluster=w585, "TrialState"=T21."Finalize", "Outcome"=enum32{"---", "Success", "Abort"}."Abort", "AbortLocation"=T20."Acq Stimulus", "AbortReason"=T19."Timed Out") -> (w586:T2)
                                n449 = local write "TrialStatus"(w586) -> ()
                                }
                                }
                              }
                              frame True {
                                n450 = local read "TrialStatus"() -> (w591:T2)
                                n451 = Bundle By Name(cluster=w591, "TrialState"=T21."Finalize", "Outcome"=enum32{"---", "Success", "Abort"}."Abort", "AbortLocation"=T20."Hold Stimulus", "AbortReason"=T19."Looked Away") -> (w592:T2)
                                n452 = local write "TrialStatus"(w592) -> ()
                              }
                            }
                          }
                        }
                      }
                      frame "TimeOut" {
                        # "Success: Save Saccade Location and Move to Finalize State"
                        n453 = local read "TrialStatus"() -> (w597:T2)
                        n454 = Bundle By Name(cluster=w597, "TrialState"=T21."Finalize", "Outcome"=enum32{"---", "Success", "Abort"}."Success", "AbortLocation"=T20."---", "AbortReason"=T19."---") -> (w600:T2)
                        n455 = Unbundle By Name(w597) -> ("StimType"=w596:enum32{"---", "Photic", "Electric"})
                        n456 = local write "TrialStatus"(w600) -> ()
                        n457 = local read "EyeXY"() -> (w595:dbl[])
                        n458 = case shown="\"Photic\", Default" w596 {
                          tunnel: w595 -> [w601 w604]
                          frame "Photic", Default {
                            n459 = local read "PhoticArray"() -> (w602:dbl[][])
                            n460 = Insert Into Array(array=w602, new element=w601) -> (w603:dbl[][])  [unwired: 2 in]
                            n461 = local write "PhoticArray"(w603) -> ()
                          }
                          frame "Electric" {
                            n462 = local read "ElectricArray"() -> (w605:dbl[][])
                            n463 = Insert Into Array(array=w605, new element=w604) -> (w606:dbl[][])  [unwired: 2 in]
                            n464 = local write "ElectricArray"(w606) -> ()
                          }
                        }
                      }
                    }
                  }
                }
                n465 = case shown="\"TimeIn\", Default" w506 {
                  frame "TimeIn", Default {
                    # "Turn On Stim and Wait"
                    n466 = call "RunOnce.vi"("Instance"=0, "Mode"=enum16{"Reset", "Run"}."Run") -> ("State"=w607:enum16{"RunOnce", "Finished"})
                    n467 = case shown="\"RunOnce\", Default" w607 {
                      frame "RunOnce", Default {
                        n468 = local read "TrialStatus"() -> (w611:T2)
                        n469 = Unbundle By Name(w611) -> ("StimType"=w610:enum32{"---", "Photic", "Electric"})
                        n470 = case shown="\"Photic\", Default" w610 {
                          frame "Photic", Default {
                            # "Turn On PStim"
                            n471 = call "SendCerebus8.vi"("String"="PStimOn" ("ASCII Data"), "Mode"=T16."String") -> ()  [unwired: 3 in]
                            n472 = local read "LEDs"() -> (w619:T7)
                            n473 = Bundle By Name(cluster=w619, "PStim"=TRUE ("LED Fixation")) -> (w618:T7)
                            n474 = local write "LEDs"(w618) -> ()
                            n475 = local read "RemoteIP"() -> (w615:u32)
                            n476 = local read "RemotePort"() -> (w614:u16)
                            n477 = local read "UDPRef"() -> (w616:refnum<k16>)
                            n478 = UDP Write(address=w615, port or service name=w614, connection ID=w616, data in="LV.ID='PStimOn';") -> ()  [unwired: 2 in, 2 out]
                          }
                          frame "Electric" {
                            # "Turn On EStim"
                            n479 = call "SendCerebus8.vi"("String"="EStimOn" ("ASCII Data"), "Mode"=T16."String") -> ()  [unwired: 3 in]
                            n480 = local read "LEDs"() -> (w628:T7)
                            n481 = Bundle By Name(cluster=w628, "EStim"=TRUE ("LED Fixation")) -> (w627:T7)
                            n482 = local write "LEDs"(w627) -> ()
                            n483 = local read "RemoteIP"() -> (w624:u32)
                            n484 = local read "UDPRef"() -> (w626:refnum<k16>)
                            n485 = local read "RemotePort"() -> (w623:u16)
                            n486 = UDP Write(address=w624, port or service name=w623, connection ID=w626, data in="LV.ID='EStimOn';") -> ()  [unwired: 2 in, 2 out]
                          }
                        }
                      }
                      frame "Finished" {
                      }
                    }
                  }
                  frame "TimeOut" {
                    # "Turn Off Stim after Waiting"
                    n487 = call "RunOnce.vi"("Instance"=1, "Mode"=enum16{"Reset", "Run"}."Run") -> ("State"=w630:enum16{"RunOnce", "Finished"})
                    n488 = case shown="\"RunOnce\", Default" w630 {
                      frame "RunOnce", Default {
                        n489 = local read "TrialStatus"() -> (w634:T2)
                        n490 = Unbundle By Name(w634) -> ("StimType"=w633:enum32{"---", "Photic", "Electric"})
                        n491 = case shown="\"Photic\", Default" w633 {
                          frame "Photic", Default {
                            # "Turn Off PStim"
                            n492 = local read "LEDs"() -> (w640:T7)
                            n493 = Bundle By Name(cluster=w640, "PStim"=FALSE ("LED Fixation")) -> (w641:T7)
                            n494 = local write "LEDs"(w641) -> ()
                            n495 = local read "RemoteIP"() -> (w636:u32)
                            n496 = local read "UDPRef"() -> (w637:refnum<k16>)
                            n497 = local read "RemotePort"() -> (w635:u16)
                            n498 = UDP Write(address=w636, port or service name=w635, connection ID=w637, data in="LV.ID='PStimOff';") -> ()  [unwired: 2 in, 2 out]
                          }
                          frame "Electric" {
                            # "This disable struct should\nbe verified!"
                            n499 = local read "LEDs"() -> (w643:T7)
                            n500 = Bundle By Name(cluster=w643, "EStim"=FALSE ("LED Fixation")) -> (w644:T7)
                            n501 = local write "LEDs"(w644) -> ()
                            n502 = disable-structure shown="Disabled" {
                              frame Disabled {
                                n503 = local read "RemoteIP"() -> (w646:u32)
                                n504 = local read "RemotePort"() -> (w645:u16)
                                n505 = local read "UDPRef"() -> (w647:refnum<k16>)
                                n506 = UDP Write(address=w646, port or service name=w645, connection ID=w647, data in="LV.ID='EStimOff';") -> ()  [unwired: 2 in, 2 out]
                              }
                              frame Enabled {
                              }
                            }
                          }
                        }
                      }
                      frame "Finished" {
                      }
                    }
                  }
                }
              }
            }
          }
          frame "Finalize" {
            n507 = case shown="\"1\"" w649 {
              tunnel: [_ _ _ _ _ _ _ _ _ _ w1171] -> w650
              frame "0" {
                w656 = FALSE ("LED Fixation")
                # "Turn off stim if stim duration exceeds time to complete a successful trial (i.e. hold fixation + hold stimulus + saccade time)."
                # "Send Appropriate Stat to MATLAB"
                n508 = local read "StimSwitchSettings"() -> (w666:T6)
                n509 = local read "TrialStatus"() -> (w668:T2)
                n510 = Unbundle By Name(w666) -> ("ElecStimMode"=w665:enum16{"Continuous", "Manual"})
                n511 = Unbundle By Name(w668) -> ("Outcome"=w667:enum32{"---", "Success", "Abort"}, "StimType"=w651:enum32{"---", "Photic", "Electric"})
                n512 = local read "TrialStatus"() -> (w658:T2)
                n513 = case shown="\"Success\"" w667 {
                  tunnel: ["LV.ID='Blank';" "LV.ID='Success';" "LV.ID='AbYBStat';"] -> w654
                  tunnel: ["---" ("ASCII Data") "Success" ("ASCII Data") "Abort" ("ASCII Data")] -> w664
                  frame "---", Default {
                  }
                  frame "Success" {
                    n514 = local read "LEDs"() -> (w680:T7)
                    n515 = Bundle By Name(cluster=w680, "Success"=TRUE ("LED Success")) -> (w679:T7)
                    n516 = local write "LEDs"(w679) -> ()
                  }
                  frame "Abort" {
                    n517 = local read "LEDs"() -> (w685:T7)
                    n518 = Bundle By Name(cluster=w685, "Abort"=TRUE ("LED Success")) -> (w684:T7)
                    n519 = local write "LEDs"(w684) -> ()
                  }
                }
                n520 = case shown="\"Manual\"" w665 {
                  tunnel: w651 -> [_ w689]
                  frame "Continuous", Default {
                  }
                  frame "Manual" {
                    n521 = case shown="\"Electric\"" w689 {
                      frame "Photic", Default {
                      }
                      frame "Electric" {
                        n522 = local write "StimButton"(FALSE ("Stim Type Button")) -> ()
                      }
                    }
                  }
                }
                n523 = case shown="\"Photic\", Default" w651 {
                  frame "Photic", Default {
                    n524 = local read "RemotePort"() -> (w669:u16)
                    n525 = local read "RemoteIP"() -> (w670:u32)
                    n526 = local read "UDPRef"() -> (w671:refnum<k16>)
                    n527 = UDP Write(address=w670, port or service name=w669, connection ID=w671, data in="LV.ID='PStimOff';") -> ()  [unwired: 2 in, 2 out]
                  }
                  frame "Electric" {
                    n528 = local read "RemotePort"() -> (w673:u16)
                    n529 = local read "RemoteIP"() -> (w674:u32)
                    n530 = local read "UDPRef"() -> (w675:refnum<k16>)
                    n531 = UDP Write(address=w674, port or service name=w673, connection ID=w675, data in="LV.ID='EStimOff';") -> ()  [unwired: 2 in, 2 out]
                  }
                }
                n532 = Unbundle By Name(w658) -> ("FinalizeState"=w657:T22)
                n533 = Increment(x=w657) -> (x+1=w659:T22)
                n534 = Bundle By Name(cluster=w658, "FinalizeState"=w659) -> (w660:T2)
                n535 = local read "RemotePort"() -> (w652:u16)
                n536 = local read "RemoteIP"() -> (w653:u32)
                n537 = local read "UDPRef"() -> (w655:refnum<k16>)
                n538 = local write "TrialStatus"(w660) -> ()
                n539 = local read "LEDs"() -> (w661:T7)
                n540 = Bundle By Name(cluster=w661, "Fixation"=w656, "PStim"=w656, "TaskInProgress"=w656, "EStim"=w656) -> (w662:T7)
                n541 = local write "LEDs"(w662) -> ()
                n542 = call "SendCerebus8.vi"("String"=w664, "Mode"=T16."String") -> ()  [unwired: 3 in]
                n543 = UDP Write(address=w653, port or service name=w652, connection ID=w655, data in=w654) -> ()  [unwired: 2 in, 2 out]
              }
              frame "1" {
                w691 = enum16{"Reset", "Run"}."Reset" ("Mode")
                w697 = enum16{"Reset", "Run"}."Reset" ("Mode")
                n544 = local read "LoopCount"() -> (w698:u64)
                n545 = local read "TrialStatus"() -> (w700:T2)
                n546 = call "LoopComp.vi"("LoopCount"=w698, "Instance"=0, "Mode"=w697) -> ()  [unwired: 3 in, 2 out]
                n547 = call "LoopComp.vi"("LoopCount"=w698, "Instance"=1, "Mode"=w697) -> ()  [unwired: 3 in, 2 out]
                n548 = Unbundle By Name(w700) -> ("FinalizeState"=w699:T22)
                n549 = Increment(x=w699) -> (x+1=w701:T22)
                n550 = call "RunOnce.vi"("Instance"=0, "Mode"=w691) -> ()  [unwired: 1 out]
                n551 = call "RunOnce.vi"("Instance"=1, "Mode"=w691) -> ()  [unwired: 1 out]
                n552 = call "RunOnce.vi"("Instance"=2, "Mode"=w691) -> ()  [unwired: 1 out]
                n553 = Bundle By Name(cluster=w700, "FinalizeState"=w701) -> (w702:T2)
                n554 = local write "TrialStatus"(w702) -> ()
              }
              frame "2" {
                # "Giving juice and acquiring waveforms"
                n555 = local read "TrialStatus"() -> (w721:T2)
                n556 = Unbundle By Name(w721) -> ("StimType"=w712:enum32{"---", "Photic", "Electric"}, "Outcome"=w711:enum32{"---", "Success", "Abort"})
                n557 = local read "Timers"() -> (w715:T12)
                n558 = Unbundle By Name(w715) -> ("ST.BRD"=w705:u64, "RT.BRD"=w720:u64)
                n559 = Equal?(x=w712, y=enum32{"---", "Photic", "Electric"}."Electric") -> (x = y?=w708:bool)
                n560 = Equal?(x=w711, y=enum32{"---", "Success", "Abort"}."Success") -> (x = y?=w707:bool)
                n561 = And(x=w708, y=w707) -> (x .and. y?=w706:bool)
                n562 = case shown="True" w706 {
                  tunnel: w705 -> [w760 w763]
                  tunnel: [w760 w761] -> w704
                  frame False {
                  }
                  frame True {
                    n563 = Multiply(x=u64 2, y=w763) -> (x*y=w761:u64)
                  }
                }
                n564 = local read "LoopPeriod"() -> (w719:u64)
                n565 = local read "LoopCount"() -> (w703:u64)
                n566 = call "LoopComp.vi"("RandTime"=w720, "LoopPeriod"=w719, "SetTime"=w704, "LoopCount"=w703, "Instance"=0, "Mode"=enum16{"Reset", "Run"}."Run") -> ("ActualTime"=w714:u64, "Outcome"=w713:enum16{"TimeIn", "TimeOut"})
                n567 = Bundle By Name(cluster=w715, "AT.BRD"=w714) -> (w716:T12)
                n568 = local write "Timers"(w716) -> ()
                n569 = case shown="\"TimeOut\"" w713 {
                  tunnel: w711 -> [w738 _]
                  frame "TimeIn", Default {
                    # "Giving Reward"
                    n570 = case shown="\"Success\"" w738 {
                      frame "---", Default {
                      }
                      frame "Success" {
                        n571 = call "RunOnce.vi"("Instance"=0, "Mode"=enum16{"Reset", "Run"}."Run") -> ("State"=w739:enum16{"RunOnce", "Finished"})
                        n572 = case shown="\"Finished\"" w739 {
                          frame "RunOnce", Default {
                            n573 = local read "LEDs"() -> (w744:T7)
                            n574 = Bundle By Name(cluster=w744, "Success"=TRUE ("LED Fixation")) -> (w743:T7)
                            n575 = local write "LEDs"(w743) -> ()
                            n576 = call-poly <vilib>:"DAQmx Write.vi"("task/channels in"=refnum<k21> "Juice", "data"=5.0) -> ()  [unwired: 11 in, 3 out]
                          }
                          frame "Finished" {
                          }
                        }
                      }
                    }
                  }
                  frame "TimeOut" {
                    n577 = local read "WfFlag"() -> (w747:bool)
                    n578 = call "RunOnce.vi"("Instance"=1, "Mode"=enum16{"Reset", "Run"}."Run") -> ("State"=w748:enum16{"RunOnce", "Finished"})
                    n579 = case shown="\"RunOnce\", Default" w748 {
                      frame "RunOnce", Default {
                        n580 = call-poly <vilib>:"DAQmx Write.vi"("task/channels in"=refnum<k21> "Juice", "data"=0.0) -> ()  [unwired: 11 in, 3 out]
                        n581 = local read "LEDs"() -> (w757:T7)
                        n582 = Bundle By Name(cluster=w757, "Success"=FALSE ("LED Fixation")) -> (w756:T7)
                        n583 = local write "LEDs"(w756) -> ()
                      }
                      frame "Finished" {
                      }
                    }
                    n584 = case shown="True" w747 {
                      frame False {
                      }
                      frame True {
                        n585 = local read "TrialStatus"() -> (w752:T2)
                        n586 = Unbundle By Name(w752) -> ("FinalizeState"=w751:T22)
                        n587 = Increment(x=w751) -> (x+1=w753:T22)
                        n588 = Bundle By Name(cluster=w752, "FinalizeState"=w753) -> (w754:T2)
                        n589 = local write "TrialStatus"(w754) -> ()
                      }
                    }
                  }
                }
                n590 = case shown="\"Electric\"" w712 {
                  frame "Photic", Default {
                    n591 = local write "WfFlag"(TRUE ("WFFlag")) -> ()
                  }
                  frame "Electric" {
                    # "Acquiring Waveforms"
                    n592 = local read "UDPRef"() -> (w725:refnum<k16>)
                    n593 = UDP Read(connection ID=w725, max size (548)=65535, timeout ms (25000)=0) -> (data out=w727:string)  [unwired: 1 in, 4 out]
                    n594 = Empty String/Path?(string/path=w727) -> (empty?=w726:bool)
                    n595 = case shown="False" w726 {
                      tunnel: w727 -> [w737 _]
                      frame False {
                        n596 = call "UDPStr2Single.vi"("UDPStr"=w737) -> ("UDPSingle"=w729:sgl[])
                        n597 = Array Size(array=w729) -> (size(s)=w730:i32)
                        n598 = Initialize Array(-0.6, w730) -> (w731:dbl[])
                        n599 = Build Array(w729, w731) -> (w734:dbl[][])
                        n600 = Bundle(-0.35, 0.04, w734) -> (w733:cluster{dbl, dbl, dbl[][]})  [unwired: 1 in]
                        n601 = local write "WfFlag"(TRUE ("WFFlag")) -> ()
                        n602 = local write "WfGraph"(w733) -> ()
                      }
                      frame True {
                      }
                    }
                  }
                }
              }
              frame "3" {
                n603 = local read "TrialStatus"() -> (w765:T2)
                n604 = Unbundle By Name(w765) -> ("FinalizeState"=w764:T22)
                n605 = Increment(x=w764) -> (x+1=w766:T22)
                n606 = Bundle By Name(cluster=w765, "FinalizeState"=w766) -> (w767:T2)
                n607 = local write "TrialStatus"(w767) -> ()
              }
              frame "4" {
                n608 = local read "TrialStatus"() -> (w768:T2)
                n609 = Unbundle By Name(w768) -> ("StimType"=w769:enum32{"---", "Photic", "Electric"})
                n610 = case shown="\"Electric\"" w769 {
                  tunnel: w768 -> [w789 w857]
                  frame "Photic", Default {
                    n611 = local read "Stats"() -> (w790:T14)
                    n612 = Unbundle By Name(w790) -> ("Photic.Total"=w784:dbl, "Photic.Successful"=w786:dbl, "Photic.HoldFixation"=w782:dbl, "Photic.AcqStimulus"=w781:dbl, "Photic.HoldStimulus"=w780:dbl, "Photic.RemovedHands"=w776:dbl)
                    n613 = Unbundle By Name(w789) -> ("Outcome"=w788:enum32{"---", "Success", "Abort"}, "AbortLocation"=w787:T20)
                    n614 = case shown="\"---\", Default" w788 {
                      tunnel: w787 -> [_ _ w817]
                      tunnel: w786 -> [w796 w804 w814]
                      tunnel: [w796 w803 w813] -> w785
                      tunnel: w784 -> [w795 w802 w816]
                      tunnel: [w795 w801 w815] -> w783
                      tunnel: w782 -> [w794 w800 w812]
                      tunnel: w781 -> [w793 w799 w811]
                      tunnel: w780 -> [w792 w798 w810]
                      tunnel: [w794 w800 w809] -> w779
                      tunnel: [w793 w799 w808] -> w778
                      tunnel: [w792 w798 w807] -> w777
                      tunnel: w776 -> [w791 w797 w806]
                      tunnel: [w791 w797 w805] -> w775
                      frame "---", Default {
                      }
                      frame "Success" {
                        n615 = Increment(x=w802) -> (x+1=w801:dbl)
                        n616 = Increment(x=w804) -> (x+1=w803:dbl)
                      }
                      frame "Abort" {
                        n617 = case shown="\"Hold Stimulus\"" w817 {
                          tunnel: w816 -> [w824 w832 w840 w848 w856]
                          tunnel: [w823 w831 w839 w845 w855] -> w815
                          tunnel: w814 -> [w822 w830 w838 w847 w854]
                          tunnel: [w822 w830 w838 w847 w854] -> w813
                          tunnel: w812 -> [w821 w829 w837 w846 w853]
                          tunnel: w811 -> [w820 w828 w835 w844 w852]
                          tunnel: w810 -> [w819 w827 w834 w842 w851]
                          tunnel: [w821 w829 w836 w846 w853] -> w809
                          tunnel: [w820 w828 w835 w843 w852] -> w808
                          tunnel: [w819 w827 w834 w842 w850] -> w807
                          tunnel: w806 -> [w818 w826 w833 w841 w849]
                          tunnel: [w818 w825 w833 w841 w849] -> w805
                          frame "---", Default {
                            n618 = Increment(x=w824) -> (x+1=w823:dbl)
                          }
                          frame "Visual Stimuli" {
                            n619 = Increment(x=w832) -> (x+1=w831:dbl)
                            n620 = Increment(x=w826) -> (x+1=w825:dbl)
                          }
                          frame "Hold Fixation" {
                            n621 = Increment(x=w840) -> (x+1=w839:dbl)
                            n622 = Increment(x=w837) -> (x+1=w836:dbl)
                          }
                          frame "Acq Stimulus" {
                            n623 = Increment(x=w848) -> (x+1=w845:dbl)
                            n624 = Increment(x=w844) -> (x+1=w843:dbl)
                          }
                          frame "Hold Stimulus" {
                            n625 = Increment(x=w856) -> (x+1=w855:dbl)
                            n626 = Increment(x=w851) -> (x+1=w850:dbl)
                          }
                        }
                      }
                    }
                    n627 = Bundle By Name(cluster=w790, "Photic.Total"=w783, "Photic.Successful"=w785, "Photic.HoldFixation"=w779, "Photic.AcqStimulus"=w778, "Photic.HoldStimulus"=w777, "Photic.RemovedHands"=w775) -> (w774:T14)
                    n628 = local write "Stats"(w774) -> ()
                  }
                  frame "Electric" {
                    n629 = local read "Stats"() -> (w873:T14)
                    n630 = Unbundle By Name(w873) -> ("Electric.Total"=w868:dbl, "Electric.Successful"=w870:dbl, "Electric.HoldFixation"=w866:dbl, "Electric.AcqStimulus"=w865:dbl, "Electric.HoldStimulus"=w864:dbl, "Electric.RemovedHands"=w860:dbl)
                    n631 = Unbundle By Name(w857) -> ("Outcome"=w872:enum32{"---", "Success", "Abort"}, "AbortLocation"=w871:T20)
                    n632 = case shown="\"Success\"" w872 {
                      tunnel: w871 -> [_ _ w900]
                      tunnel: w870 -> [w879 w887 w897]
                      tunnel: [w879 w886 w896] -> w869
                      tunnel: w868 -> [w878 w885 w899]
                      tunnel: [w878 w884 w898] -> w867
                      tunnel: w866 -> [w877 w883 w895]
                      tunnel: w865 -> [w876 w882 w894]
                      tunnel: w864 -> [w875 w881 w893]
                      tunnel: [w877 w883 w892] -> w863
                      tunnel: [w876 w882 w891] -> w862
                      tunnel: [w875 w881 w890] -> w861
                      tunnel: w860 -> [w874 w880 w889]
                      tunnel: [w874 w880 w888] -> w859
                      frame "---", Default {
                      }
                      frame "Success" {
                        n633 = Increment(x=w885) -> (x+1=w884:dbl)
                        n634 = Increment(x=w887) -> (x+1=w886:dbl)
                      }
                      frame "Abort" {
                        n635 = case shown="\"Visual Stimuli\"" w900 {
                          tunnel: w899 -> [w907 w915 w923 w931 w939]
                          tunnel: [w906 w914 w922 w928 w938] -> w898
                          tunnel: w897 -> [w905 w913 w921 w930 w937]
                          tunnel: [w905 w913 w921 w930 w937] -> w896
                          tunnel: w895 -> [w904 w912 w920 w929 w936]
                          tunnel: w894 -> [w903 w911 w918 w927 w935]
                          tunnel: w893 -> [w902 w910 w917 w925 w934]
                          tunnel: [w904 w912 w919 w929 w936] -> w892
                          tunnel: [w903 w911 w918 w926 w935] -> w891
                          tunnel: [w902 w910 w917 w925 w933] -> w890
                          tunnel: w889 -> [w901 w909 w916 w924 w932]
                          tunnel: [w901 w908 w916 w924 w932] -> w888
                          frame "---", Default {
                            n636 = Increment(x=w907) -> (x+1=w906:dbl)
                          }
                          frame "Visual Stimuli" {
                            n637 = Increment(x=w915) -> (x+1=w914:dbl)
                            n638 = Increment(x=w909) -> (x+1=w908:dbl)
                          }
                          frame "Hold Fixation" {
                            n639 = Increment(x=w923) -> (x+1=w922:dbl)
                            n640 = Increment(x=w920) -> (x+1=w919:dbl)
                          }
                          frame "Acq Stimulus" {
                            n641 = Increment(x=w931) -> (x+1=w928:dbl)
                            n642 = Increment(x=w927) -> (x+1=w926:dbl)
                          }
                          frame "Hold Stimulus" {
                            n643 = Increment(x=w939) -> (x+1=w938:dbl)
                            n644 = Increment(x=w934) -> (x+1=w933:dbl)
                          }
                        }
                      }
                    }
                    n645 = Bundle By Name(cluster=w873, "Electric.Total"=w867, "Electric.Successful"=w869, "Electric.HoldFixation"=w863, "Electric.AcqStimulus"=w862, "Electric.HoldStimulus"=w861, "Electric.RemovedHands"=w859) -> (w858:T14)
                    n646 = local write "Stats"(w858) -> ()
                  }
                }
                n647 = local read "TrialStatus"() -> (w771:T2)
                n648 = Unbundle By Name(w771) -> ("FinalizeState"=w770:T22)
                n649 = Increment(x=w770) -> (x+1=w772:T22)
                n650 = Bundle By Name(cluster=w771, "FinalizeState"=w772) -> (w773:T2)
                n651 = local write "TrialStatus"(w773) -> ()
              }
              frame "5" {
                # "Edited it to handle BGnd from the Matlab Command"
                # "This subvi needs work!!!"
                n652 = local read "TrialStatus"() -> (w950:T2)
                n653 = local read "EyeCalibration"() -> (w944:T15)
                n654 = local read "MATLABCom"() -> (w947:string)
                n655 = local read "TrialStatus"() -> (w943:T2)
                n656 = local read "Timers"() -> (w946:T12)
                n657 = Unbundle By Name(w950) -> ("FinalizeState"=w949:T22)
                n658 = local read "LoopCount"() -> (w940:u64)
                n659 = call "CerebusParamsCom.vi"("EyeCalibration"=w944, "MatlabCommand"=w947, "Timers"=w946, "TrialStatus"=w943) -> ("CerebusCommand"=w945:string)
                n660 = Increment(x=w949) -> (x+1=w951:T22)
                n661 = Bundle By Name(cluster=w950, "FinalizeState"=w951) -> (w952:T2)
                n662 = call "LoopComp.vi"("LoopCount"=w940, "Instance"=0, "Mode"=enum16{"Reset", "Run"}."Reset") -> ()  [unwired: 3 in, 2 out]
                n663 = call "SendCerebus8.vi"("String"=w945, "Mode"=T16."String") -> ()  [unwired: 3 in]
                n664 = local write "TrialStatus"(w952) -> ()
              }
              frame "6" {
                # "Penalty"
                n665 = local read "TrialStatus"() -> (w954:T2)
                n666 = Unbundle By Name(w954) -> ("Outcome"=w953:enum32{"---", "Success", "Abort"})
                n667 = case shown="\"---\", Default" w953 {
                  frame "---", Default {
                    w955 = enum16{"Reset", "Run"}."Reset" ("Mode")
                    w961 = enum16{"Reset", "Run"}."Reset" ("Mode")
                    n668 = local read "TrialStatus"() -> (w964:T2)
                    n669 = local read "LoopCount"() -> (w962:u64)
                    n670 = Unbundle By Name(w964) -> ("FinalizeState"=w963:T22)
                    n671 = call "LoopComp.vi"("LoopCount"=w962, "Instance"=0, "Mode"=w961) -> ()  [unwired: 3 in, 2 out]
                    n672 = call "LoopComp.vi"("LoopCount"=w962, "Instance"=1, "Mode"=w961) -> ()  [unwired: 3 in, 2 out]
                    n673 = Increment(x=w963) -> (x+1=w965:T22)
                    n674 = Bundle By Name(cluster=w964, "FinalizeState"=w965) -> (w966:T2)
                    n675 = call "RunOnce.vi"("Instance"=0, "Mode"=w955) -> ()  [unwired: 1 out]
                    n676 = call "RunOnce.vi"("Instance"=1, "Mode"=w955) -> ()  [unwired: 1 out]
                    n677 = call "RunOnce.vi"("Instance"=2, "Mode"=w955) -> ()  [unwired: 1 out]
                    n678 = local write "TrialStatus"(w966) -> ()
                  }
                  frame "Abort" {
                    n679 = local read "Timers"() -> (w970:T12)
                    n680 = local read "LoopPeriod"() -> (w976:u64)
                    n681 = local read "LoopCount"() -> (w967:u64)
                    n682 = Unbundle By Name(w970) -> ("ST.FPD"=w973:u64, "RT.FPD"=w971:u64)
                    n683 = call "LoopComp.vi"("RandTime"=w971, "LoopPeriod"=w976, "SetTime"=w973, "LoopCount"=w967, "Instance"=0, "Mode"=enum16{"Reset", "Run"}."Run") -> ("ActualTime"=w969:u64, "Outcome"=w972:enum16{"TimeIn", "TimeOut"})
                    n684 = Bundle By Name(cluster=w970, "AT.FPD"=w969) -> (w968:T12)
                    n685 = local write "Timers"(w968) -> ()
                    n686 = case shown="\"TimeOut\"" w972 {
                      frame "TimeIn", Default {
                      }
                      frame "TimeOut" {
                        w977 = enum16{"Reset", "Run"}."Reset" ("Mode")
                        w982 = enum16{"Reset", "Run"}."Reset" ("Mode")
                        n687 = local read "TrialStatus"() -> (w985:T2)
                        n688 = local read "LoopCount"() -> (w983:u64)
                        n689 = Unbundle By Name(w985) -> ("FinalizeState"=w984:T22)
                        n690 = call "LoopComp.vi"("LoopCount"=w983, "Instance"=0, "Mode"=w982) -> ()  [unwired: 3 in, 2 out]
                        n691 = call "LoopComp.vi"("LoopCount"=w983, "Instance"=1, "Mode"=w982) -> ()  [unwired: 3 in, 2 out]
                        n692 = Increment(x=w984) -> (x+1=w986:T22)
                        n693 = Bundle By Name(cluster=w985, "FinalizeState"=w986) -> (w987:T2)
                        n694 = call "RunOnce.vi"("Instance"=0, "Mode"=w977) -> ()  [unwired: 1 out]
                        n695 = call "RunOnce.vi"("Instance"=1, "Mode"=w977) -> ()  [unwired: 1 out]
                        n696 = local write "TrialStatus"(w987) -> ()
                      }
                    }
                  }
                }
              }
              frame "7" {
                # "Pause"
                n697 = local read "Global Controls"() -> (w989:T11)
                n698 = Unbundle By Name(w989) -> ("Pause"=w988:bool)
                n699 = case shown="True" w988 {
                  frame False {
                    n700 = local read "TrialStatus"() -> (w991:T2)
                    n701 = Unbundle By Name(w991) -> ("FinalizeState"=w990:T22)
                    n702 = Increment(x=w990) -> (x+1=w992:T22)
                    n703 = Bundle By Name(cluster=w991, "FinalizeState"=w992) -> (w993:T2)
                    n704 = local write "TrialStatus"(w993) -> ()
                  }
                  frame True {
                    n705 = local read "PauseControls"() -> (w999:T10)
                    n706 = Unbundle By Name(w999) -> ("FixationTime"=w994:dbl, "Fixate"=w998:bool, "Stimulate"=w997:bool, "StimLoad"=w996:bool, "PauseType"=w995:bool)
                    n707 = case shown="True" w997 {
                      tunnel: w995 -> [_ w1025]
                      frame False {
                        w1019 = enum16{"Reset", "Run"}."Reset" ("Mode")
                        n708 = local read "LoopCount"() -> (w1024:u64)
                        n709 = call "LoopComp.vi"("LoopCount"=w1024, "Instance"=1, "Mode"=enum16{"Reset", "Run"}."Reset") -> ()  [unwired: 3 in, 2 out]
                        n710 = call "RunOnce.vi"("Instance"=1, "Mode"=w1019) -> ()  [unwired: 1 out]
                        n711 = call "RunOnce.vi"("Instance"=2, "Mode"=w1019) -> ()  [unwired: 1 out]
                      }
                      frame True {
                        n712 = case shown="False" w1025 {
                          frame False {
                            n713 = local read "Timers"() -> (w1030:T12)
                            n714 = local read "LoopPeriod"() -> (w1027:u64)
                            n715 = local read "LoopCount"() -> (w1026:u64)
                            n716 = Unbundle By Name(w1030) -> ("ST.SD"=w1031:u64)
                            n717 = call "LoopComp.vi"("LoopPeriod"=w1027, "SetTime"=w1031, "LoopCount"=w1026, "Instance"=1, "Mode"=enum16{"Reset", "Run"}."Run") -> ("Outcome"=w1029:enum16{"TimeIn", "TimeOut"})  [unwired: 1 in, 1 out]
                            n718 = case shown="\"TimeOut\"" w1029 {
                              frame "TimeIn", Default {
                                n719 = call "RunOnce.vi"("Instance"=1, "Mode"=enum16{"Reset", "Run"}."Run") -> ("State"=w1035:enum16{"RunOnce", "Finished"})
                                n720 = case shown="\"Finished\"" w1035 {
                                frame "RunOnce", Default {
                                n721 = local read "RemotePort"() -> (w1036:u16)
                                n722 = local read "RemoteIP"() -> (w1037:u32)
                                n723 = local read "UDPRef"() -> (w1039:refnum<k16>)
                                n724 = UDP Write(address=w1037, port or service name=w1036, connection ID=w1039, data in="LV.ID='PStimOn';") -> ()  [unwired: 2 in, 2 out]
                                }
                                frame "Finished" {
                                }
                                }
                              }
                              frame "TimeOut" {
                                n725 = local read "PauseControls"() -> (w1044:T10)
                                n726 = Bundle By Name(cluster=w1044, "Stimulate"=FALSE ("Show Fixation")) -> (w1045:T10)
                                n727 = local write "PauseControls"(w1045) -> ()
                                n728 = local read "RemotePort"() -> (w1043:u16)
                                n729 = local read "RemoteIP"() -> (w1042:u32)
                                n730 = local read "UDPRef"() -> (w1041:refnum<k16>)
                                n731 = UDP Write(address=w1042, port or service name=w1043, connection ID=w1041, data in="LV.ID='PStimOff';") -> ()  [unwired: 2 in, 2 out]
                              }
                            }
                          }
                          frame True {
                            n732 = call "RunOnce.vi"("Instance"=2, "Mode"=enum16{"Reset", "Run"}."Run") -> ("State"=w1049:enum16{"RunOnce", "Finished"})
                            n733 = case shown="\"Finished\"" w1049 {
                              frame "RunOnce", Default {
                                n734 = local read "RemotePort"() -> (w1053:u16)
                                n735 = local read "RemoteIP"() -> (w1052:u32)
                                n736 = local read "UDPRef"() -> (w1051:refnum<k16>)
                                n737 = UDP Write(address=w1052, port or service name=w1053, connection ID=w1051, data in="LV.ID='EStimOn';") -> ()  [unwired: 2 in, 2 out]
                              }
                              frame "Finished" {
                                n738 = local read "UDPRef"() -> (w1056:refnum<k16>)
                                n739 = UDP Read(connection ID=w1056, max size (548)=65535, timeout ms (25000)=0) -> (data out=w1058:string)  [unwired: 1 in, 4 out]
                                n740 = Empty String/Path?(string/path=w1058) -> (empty?=w1057:bool)
                                n741 = case shown="False" w1057 {
                                tunnel: w1058 -> [w1070 _]
                                frame False {
                                n742 = call "UDPStr2Single.vi"("UDPStr"=w1070) -> ("UDPSingle"=w1062:sgl[])
                                n743 = Array Size(array=w1062) -> (size(s)=w1063:i32)
                                n744 = Initialize Array(-0.6, w1063) -> (w1064:dbl[])
                                n745 = Build Array(w1062, w1064) -> (w1067:dbl[][])
                                n746 = Bundle(-0.35, 0.04, w1067) -> (w1066:cluster{dbl, dbl, dbl[][]})  [unwired: 1 in]
                                n747 = local write "WfGraph"(w1066) -> ()
                                n748 = local read "PauseControls"() -> (w1059:T10)
                                n749 = Bundle By Name(cluster=w1059, "Stimulate"=FALSE ("Show Fixation")) -> (w1060:T10)
                                n750 = local write "PauseControls"(w1060) -> ()
                                }
                                frame True {
                                }
                                }
                              }
                            }
                          }
                        }
                      }
                    }
                    n751 = case shown="True" w998 {
                      tunnel: w994 -> [_ w1077]
                      frame False {
                        n752 = local read "LoopCount"() -> (w1071:u64)
                        n753 = call "LoopComp.vi"("LoopCount"=w1071, "Instance"=0, "Mode"=enum16{"Reset", "Run"}."Reset") -> ()  [unwired: 3 in, 2 out]
                      }
                      frame True {
                        n754 = local read "LoopPeriod"() -> (w1075:u64)
                        n755 = local read "LoopCount"() -> (w1074:u64)
                        n756 = call "LoopComp.vi"("LoopPeriod"=w1075, "SetTime"=w1077, "LoopCount"=w1074, "Instance"=0, "Mode"=enum16{"Reset", "Run"}."Run") -> ("Outcome"=w1078:enum16{"TimeIn", "TimeOut"})  [unwired: 1 in, 1 out]
                        n757 = case shown="\"TimeOut\"" w1078 {
                          frame "TimeIn", Default {
                            n758 = call "RunOnce.vi"("Instance"=0, "Mode"=enum16{"Reset", "Run"}."Run") -> ("State"=w1080:enum16{"RunOnce", "Finished"})
                            n759 = case shown="\"Finished\"" w1080 {
                              frame "RunOnce", Default {
                                n760 = local read "PauseControls"() -> (w1087:T10)
                                n761 = Bundle By Name(cluster=w1087, "Fixate"=TRUE ("Show Fixation")) -> (w1088:T10)
                                n762 = local write "PauseControls"(w1088) -> ()
                                n763 = local read "RemoteIP"() -> (w1084:u32)
                                n764 = local read "RemotePort"() -> (w1083:u16)
                                n765 = local read "UDPRef"() -> (w1085:refnum<k16>)
                                n766 = UDP Write(address=w1084, port or service name=w1083, connection ID=w1085, data in="LV.ID='FixOn';") -> ()  [unwired: 2 in, 2 out]
                              }
                              frame "Finished" {
                              }
                            }
                          }
                          frame "TimeOut" {
                            n767 = local read "RemotePort"() -> (w1092:u16)
                            n768 = local read "UDPRef"() -> (w1095:refnum<k16>)
                            n769 = local read "RemoteIP"() -> (w1093:u32)
                            n770 = call "RunOnce.vi"("Instance"=0, "Mode"=enum16{"Reset", "Run"}."Reset") -> ()  [unwired: 1 out]
                            n771 = UDP Write(address=w1093, port or service name=w1092, connection ID=w1095, data in="LV.ID='FixOff';") -> ()  [unwired: 2 in, 2 out]
                            n772 = local read "PauseControls"() -> (w1096:T10)
                            n773 = Bundle By Name(cluster=w1096, "Fixate"=FALSE ("Show Fixation")) -> (w1097:T10)
                            n774 = local write "PauseControls"(w1097) -> ()
                          }
                        }
                      }
                    }
                    n775 = case shown="True" w996 {
                      tunnel: w995 -> [_ w1006]
                      frame False {
                      }
                      frame True {
                        n776 = case shown="False" w1006 {
                          tunnel: [w1014 w1017] -> w1004
                          frame False {
                            n777 = local read "TrialStatus"() -> (w1015:T2)
                            n778 = Bundle By Name(cluster=w1015, "StimType"=enum32{"---", "Photic", "Electric"}."Photic") -> (w1014:T2)
                          }
                          frame True {
                            n779 = local read "TrialStatus"() -> (w1018:T2)
                            n780 = Bundle By Name(cluster=w1018, "StimType"=enum32{"---", "Photic", "Electric"}."Electric") -> (w1017:T2)
                          }
                        }
                        n781 = local read "PhoticStimSettings"() -> (w1007:T13)
                        n782 = local read "ElecStimSettings"() -> (w1005:T1)
                        n783 = local read "Electrodes"() -> (w1009:T9)
                        n784 = call "MatlabStimCom.vi"("TrialStatus"=w1004, "PhoticStimSettings"=w1007, "ElecStimSettings"=w1005, "Electrodes"=w1009) -> ("MATLABCom"=w1000:string, "Current Electrode"=w1008:i32)  [unwired: 1 in]
                        n785 = local write "Current Electrode"(w1008) -> ()
                        n786 = local write "MATLABCom"(w1000) -> ()
                        n787 = local read "RemotePort"() -> (w1003:u16)
                        n788 = local read "RemoteIP"() -> (w1002:u32)
                        n789 = local read "UDPRef"() -> (w1001:refnum<k16>)
                        n790 = UDP Write(address=w1002, port or service name=w1003, connection ID=w1001, data in=w1000) -> ()  [unwired: 2 in, 2 out]
                        n791 = local read "PauseControls"() -> (w1010:T10)
                        n792 = Bundle By Name(cluster=w1010, "StimLoad"=FALSE ("Show Fixation")) -> (w1011:T10)
                        n793 = local write "PauseControls"(w1011) -> ()
                      }
                    }
                  }
                }
              }
              frame "8" {
                n794 = local read "TrialStatus"() -> (w1100:T2)
                n795 = Unbundle By Name(w1100) -> ("FinalizeState"=w1099:T22)
                n796 = Increment(x=w1099) -> (x+1=w1101:T22)
                n797 = Bundle By Name(cluster=w1100, "FinalizeState"=w1101) -> (w1102:T2)
                n798 = local write "TrialStatus"(w1102) -> ()
              }
              frame "9" {
                # "Reset plots and send comments"
                n799 = local read "Global Controls"() -> (w1112:T11)
                n800 = Unbundle By Name(w1112) -> ("PhoticReset"=w1111:bool, "ElecReset"=w1110:bool, "Comment"=w1109:bool)
                n801 = Build Array(w1111, w1110, w1109) -> (w1108:bool[])
                n802 = local read "TrialStatus"() -> (w1104:T2)
                n803 = Or Array Elements(Boolean array=w1108) -> (logical OR=w1107:bool)
                n804 = case shown="True" w1107 {
                  frame False {
                  }
                  frame True {
                    n805 = stacked-sequence {
                      frame #0 {
                        n806 = local read "RemotePort"() -> (w1113:u16)
                        n807 = local read "RemoteIP"() -> (w1114:u32)
                        n808 = local read "UDPRef"() -> (w1115:refnum<k16>)
                        n809 = UDP Write(address=w1114, port or service name=w1113, connection ID=w1115, data in="LV.ID='Blank';" ("write buffer")) -> ()  [unwired: 2 in, 2 out]
                        n810 = call-poly <vilib>:"DAQmx Write.vi"("task/channels in"=refnum<k21> "Juice", "data"=0.0) -> ()  [unwired: 11 in, 3 out]
                      }
                      frame #1 {
                        n811 = local read "Global Controls"() -> (w1120:T11)
                        n812 = Unbundle By Name(w1120) -> ("Comment"=w1119:bool)
                        n813 = case shown="True" w1119 {
                          frame False {
                          }
                          frame True {
                            n814 = stacked-sequence {
                              frame #0 {
                                n815 = local read "Comments"() -> (w1125:string)
                                n816 = Concatenate Strings("Comments:Comments=" ("Key Word"), w1125, ";" ("Key Word")) -> (w1121:string)
                                n817 = call "SendCerebus8.vi"("String"=w1121, "Mode"=T16."String") -> ()  [unwired: 3 in]
                              }
                              frame #1 {
                                n818 = local read "Comments"() -> (w1127:string)
                                n819 = local read "Database"() -> (w1131:T3)
                                n820 = Unbundle By Name(w1131) -> ("TaskComments"=w1129:string)
                                n821 = call <vilib>:"Trim Whitespace.vi"("string"=w1129) -> ("trimmed string"=w1128:string)  [unwired: 1 in]
                                n822 = call <vilib>:"Trim Whitespace.vi"("string"=w1127) -> ("trimmed string"=w1126:string)  [unwired: 1 in]
                                n823 = Concatenate Strings(w1128, "\r", w1126) -> (w1133:string)
                                n824 = Bundle By Name(cluster=w1131, "TaskComments"=w1133) -> (w1132:T3)
                                n825 = local write "Database"(w1132) -> ()
                              }
                              frame #2 {
                                n826 = local read "Global Controls"() -> (w1135:T11)
                                n827 = Bundle By Name(cluster=w1135, "Comment"=FALSE ("RESET")) -> (w1136:T11)
                                n828 = local write "Global Controls"(w1136) -> ()
                              }
                            }
                          }
                        }
                      }
                      frame #2 {
                        n829 = local read "Global Controls"() -> (w1138:T11)
                        n830 = Unbundle By Name(w1138) -> ("PhoticReset"=w1137:bool)
                        n831 = case shown="True" w1137 {
                          frame False {
                          }
                          frame True {
                            n832 = local read "Stats"() -> (w1140:T14)
                            n833 = call "SendCerebus8.vi"("String"="PhoticReset" ("ASCII Data"), "Mode"=T16."String") -> ()  [unwired: 3 in]
                            n834 = Bundle By Name(cluster=w1140, "Photic"=T23 {"AcqStimulus"=0.0, "HoldStimulus"=0.0, "HoldFixation"=0.0, "Successful"=0.0, "Total"=0.0, "RemovedHands"=0.0}) -> (w1141:T14)
                            n835 = local write "PhoticArray"(dbl[][] [] ("initialized array")) -> ()
                            n836 = local read "Global Controls"() -> (w1148:T11)
                            n837 = local write "Stats"(w1141) -> ()
                            n838 = Bundle By Name(cluster=w1148, "PhoticReset"=FALSE ("Photic Reset"), "Pause"=TRUE) -> (w1147:T11)
                            n839 = local write "Global Controls"(w1147) -> ()
                          }
                        }
                      }
                      frame #3 {
                        n840 = local read "Global Controls"() -> (w1150:T11)
                        n841 = Unbundle By Name(w1150) -> ("ElecReset"=w1149:bool)
                        n842 = case shown="True" w1149 {
                          frame False {
                          }
                          frame True {
                            n843 = call "SendCerebus8.vi"("String"="ElectricReset" ("ASCII Data"), "Mode"=T16."String") -> ()  [unwired: 3 in]
                            n844 = local read "Stats"() -> (w1154:T14)
                            n845 = Bundle By Name(cluster=w1154, "Electric"=T23 {"AcqStimulus"=0.0, "HoldStimulus"=0.0, "HoldFixation"=0.0, "Successful"=0.0, "Total"=0.0, "RemovedHands"=0.0} ("Photic")) -> (w1153:T14)
                            n846 = local write "ElectricArray"(dbl[][] [] ("initialized array")) -> ()
                            n847 = local read "Global Controls"() -> (w1159:T11)
                            n848 = local write "Stats"(w1153) -> ()
                            n849 = Bundle By Name(cluster=w1159, "ElecReset"=FALSE ("Elec Reset"), "Pause"=TRUE ("Photic Reset")) -> (w1160:T11)
                            n850 = local write "Global Controls"(w1160) -> ()
                          }
                        }
                      }
                    }
                  }
                }
                n851 = Unbundle By Name(w1104) -> ("FinalizeState"=w1103:T22)
                n852 = Increment(x=w1103) -> (x+1=w1105:T22)
                n853 = Bundle By Name(cluster=w1104, "FinalizeState"=w1105) -> (w1106:T2)
                n854 = local write "TrialStatus"(w1106) -> ()
              }
              frame "10" {
                w1168 = FALSE ("LED Fixation")
                w1173 = FALSE ("Stimulate")
                # "Restart"
                n855 = local read "PauseControls"() -> (w1175:T10)
                n856 = Bundle By Name(cluster=w1175, "Stimulate"=w1173, "StimLoad"=w1173, "Fixate"=w1173, "PauseType"=w1173) -> (w1174:T10)
                n857 = local read "TrialStatus"() -> (w1166:T2)
                n858 = Bundle By Name(cluster=w1166, "TrialState"=T21."Initialize", "InitializeState"=T22."0", "FinalizeState"=T22."0") -> (w1167:T2)
                n859 = local write "PauseControls"(w1174) -> ()
                n860 = call-poly <vilib>:"DAQmx Write.vi"("task/channels in"=refnum<k21> "Juice", "data"=0.0) -> ()  [unwired: 11 in, 3 out]
                n861 = local write "TrialStatus"(w1167) -> ()
                n862 = local read "Global Controls"() -> (w1172:T11)
                n863 = Unbundle By Name(w1172) -> ("Stop"=w1171:bool)
                n864 = local read "LEDs"() -> (w1169:T7)
                n865 = Bundle By Name(cluster=w1169, "Success"=w1168, "Failure"=w1168, "Abort"=w1168) -> (w1170:T7)
                n866 = local write "LEDs"(w1170) -> ()
              }
            }
          }
        }
        n867 = node-c288() -> ()  [unwired: 1 out]
        "LoopCount" <- w166
      }
      n868 = node-c288(w133) -> ()
    }
    frame #2 {
      n869 = stacked-sequence {
        frame #0 {
          # "Also add window resizing"
        }
        frame #1 {
          n870 = disable-structure shown="Disabled" {
            frame Disabled {
              n871 = local read "ExperimentDate"() -> (w1193:timestamp)
              n872 = local read "CerebusFolder"() -> (w1190:string)
              n873 = local read "TaskType"() -> (w1192:string)
              n874 = local read "Database"() -> (w1194:T3)
              n875 = Empty String/Path?(string/path=w1190) -> (empty?=w1191:bool)
              n876 = Bundle By Name(cluster=w1194, "ExperimentDate"=w1193, "CerebusFolder"=w1190, "TaskType"=w1192) -> (w1188:T3)
              n877 = case shown="True" w1191 {
                frame False {
                }
                frame True {
                  n878 = One Button Dialog(message="The Cerebus data folder is unknown\nand will not be saved to the database.\nMake sure to update the database\nmanually with the appropriate folder\nname!") -> ()  [unwired: 1 in, 1 out]
                }
              }
              n879 = local write "Database"(w1188) -> ()
              n880 = call "UpdateDatabaseRemote.vi"("DatabaseIn"=w1188, "CallType"=enum16{"Initialize", "Save", "Load"}."Save") -> ()  [unwired: 1 in, 3 out]
              n881 = call "SendDatabase2Cerebus.vi"("Database"=w1188) -> ()  [unwired: 1 out]
            }
            frame Enabled {
            }
          }
        }
        frame #2 {
          # "Stop Cerebus recording"
          n882 = local read "StopRecording"() -> (w1196:bool)
          n883 = case shown="True" w1196 {
            frame False {
            }
            frame True {
              n884 = local read "AutoCentraVI"() -> (w1198:path)
              n885 = Open Application Reference(10:u16 3362 ("port number or service name (3363)"), 11:"155.101.184.11" ("machine name (\"\":  open local reference)")) -> (0:w1201:errorcluster, 3:w1203:refnum<vi>)  [unwired: 2 in]
              n886 = Open VI Reference(type specifier VI Refnum (for type only)=refnum<vi> refnum, application reference (local)=w1203, vi path=w1198, error in (no error)=w1201) -> (vi reference=w1199:refnum<vi>, error out=w1200:errorcluster)  [unwired: 2 in]
              n887 = call-by-ref "?"(reference=w1199, error in=w1200, "Mode"=T17."StopRecording") -> ("Recording?"=w1197:bool)  [unwired: 2 in, 4 out]
              n888 = local write "Recording?"(w1197) -> ()
            }
          }
        }
        frame #3 {
          n889 = local read "RemotePort"() -> (w1221:u16)
          n890 = local read "RemoteIP"() -> (w1220:u32)
          n891 = local read "UDPRef"() -> (w1222:refnum<k16>)
          n892 = local read "Global Controls"() -> (w1218:T11)
          n893 = UDP Write(address=w1220, port or service name=w1221, connection ID=w1222, data in="LV.ID='ExitProgram';" ("write buffer")) -> (error out=w1211:errorcluster, 3:w1212:refnum<k16>)  [unwired: 2 in]
          n894 = Bundle By Name(cluster=w1218, "Stop"=FALSE ("LED Fixation")) -> (w1219:T11)
          n895 = local write "Global Controls"(w1219) -> ()
          n896 = UDP Close(connection ID=w1212, 8:w1211) -> ()  [unwired: 2 out]
          n897 = call "SendCerebus8.vi"("Mode"=T16."Close") -> ()  [unwired: 4 in]
          n898 = local write "LEDs"(T7 {"InRange"=FALSE, "TaskInProgress"=FALSE, "Fixation"=FALSE, "PStim"=FALSE, "Success"=FALSE, "Failure"=FALSE, "Abort"=FALSE, "HandsReady"=FALSE, "RightHand"=FALSE, "LeftHand"=FALSE, "EStim"=FALSE} ("LEDs")) -> ()
          n899 = disable-structure shown="Disabled" {
            frame Disabled {
              # "TF = start recording\nFT = stop recording\nTT = stop recording\nFF = initialize"
              n900 = Build Array(TRUE, TRUE) -> (w1225:bool[])
              n901 = call-poly <vilib>:"DAQmx Write.vi"("task/channels in"=refnum<k21> "Cerebus2Trig", "data"=w1225) -> ()  [unwired: 11 in, 3 out]
            }
            frame Enabled {
            }
          }
          n902 = call "EyeTracker.vi"("Mode"=enum16{"Initialize", "Run", "Close"}."Close") -> ()  [unwired: 1 out]
          n903 = call "ReadCapacitanceSwitches.vi"("Mode"=enum32{"Initialize", "Run", "Close"}."Close") -> ()  [unwired: 3 out]
          n904 = call-poly <vilib>:"DAQmx Write.vi"("task/channels in"=refnum<k21> "Juice", "data"=0.0) -> ("task out"=w1208:refnum<k21>, "error out"=w1207:errorcluster)  [unwired: 11 in, 1 out]
          n905 = call <vilib>:"DAQmx Stop Task.vi"("task/channels in"=w1208, "error in"=w1207) -> ("error out"=w1213:errorcluster)  [unwired: 12 in, 1 out]
          n906 = call <vilib>:"Simple Error Handler.vi"("error in (no error)"=w1213) -> ()  [unwired: 4 in, 5 out]
        }
      }
    }
  }
